vi "Defect Buddy 2014-11-16.vi"() -> ()   [LabVIEW 2010]
uses:
  <vilib>/addons/database/_DB Variant To Data/Database Variant To Data.xnode
  <vilib>/addons/database/NI_Database_API.lvlib
  <vilib>/picture/3D Picture Control/NI_3D Picture Control.lvlib
  <vilib>/Utility/file.llb/Write To Spreadsheet File (string).vi
  <vilib>/addons/database/Connection.llb/Conn Execute.vi
  <vilib>/addons/database/Recordset.llb/Rec Destroy - Connection.vi
  <vilib>/addons/database/Recordset.llb/Rec Fetch Recordset Data (R).vi
  <vilib>/addons/database/Connection.llb/DB Tools Open Connec (Path).vi
  <vilib>/addons/database/Connection.llb/Conn ObjectReference.ctl
panel:
  out "Separate Defects":cluster{i32, i32}[](array[cluster])
  in  "Bound Pairs":T1(array[cluster])
  out "element 2":cluster{i32, i32}
  out "element":cluster{i32, i32}
  out "Array 2":T2(array[cluster])
  out "Array":string[][](array[string])
  out "spreadsheet string":string
  in  "Volumes":dbl[](array[numeric])=[5230.5515143, 4360.60278, 2309.371815, 7792.576126]
  in  "Markov-Payne Correction":bool
  out "Loaded Structure":T3={"Structure Name"="Batch6_3+111 Quasi-Bulk", "Lattice vector a"=[9.1641, 0.0, 0.0], "Lattice vector b"=[0.0, 7.93635, 0.0], "Lattice vector c"=[0.0, 0.0, 53.7091], "Atoms Array"=[{"Atom Name"="", "Positions (Direct)"=[[0.036896, 0.129554, 0.035254], [0.536896, 0.129554, 0.035254], [0.286896, 0.629554, 0.035254], [0.786896, 0.629554, 0.035254], [0.285415, 0.295133, 0.107673], [0.785415, 0.295133, 0.107673], [0.035415, 0.795133, 0.107673], [0.535415, 0.795133, 0.107673], [0.033615, 0.463308, 0.180101], [0.533615, 0.463308, 0.180101], [0.283615, 0.963308, 0.180101], [0.783615, 0.963308, 0.180101], [0.030844, 0.131453, 0.252535], [0.530844, 0.131453, 0.252535], [0.280844, 0.631453, 0.252535], [0.780844, 0.631453, 0.252535], [0.278379, 0.302058, 0.324923], [0.778379, 0.302058, 0.324923], [0.028379, 0.802058, 0.324923], [0.528379, 0.802058, 0.324923], [0.031198, 0.471844, 0.397363], [0.531198, 0.471844, 0.397363], [0.281198, 0.971844, 0.397363], [0.781198, 0.971844, 0.397363], [0.03247, 0.140643, 0.469814], [0.53247, 0.140643, 0.469814], [0.28247, 0.640643, 0.469814], [0.78247, 0.640643, 0.469814], [0.284308, 0.303948, 0.542263], [0.784308, 0.303948, 0.542263], [0.034308, 0.803948, 0.542263], [0.534308, 0.803948, 0.542263], [0.035944, 0.468219, 0.614701], [0.535944, 0.468219, 0.614701], [0.285944, 0.968219, 0.614701], [0.785944, 0.968219, 0.614701], [0.037813, 0.131858, 0.687216], [0.537813, 0.131858, 0.687216], [0.787813, 0.631858, 0.687216], [0.287813, 0.631858, 0.687216], [0.038238, 0.463759, 0.759817], [0.538238, 0.463759, 0.759817], [0.288238, 0.963758, 0.759817], [0.788238, 0.963758, 0.759817], [0.038639, 0.130134, 0.831025], [0.538639, 0.130134, 0.831025], [0.288639, 0.630134, 0.831025], [0.788639, 0.630134, 0.831025], [0.285712, 0.295024, 0.89873], [0.785712, 0.295024, 0.89873], [0.035712, 0.795024, 0.89873], [0.535712, 0.795024, 0.89873], [0.032596, 0.464879, 0.966384], [0.532596, 0.464879, 0.966384], [0.282596, 0.964879, 0.966384], [0.782596, 0.964879, 0.966384]], "Positions (Cartesian)"=[[0.33811863359999994, 1.0281858879, 1.8934606114], [4.9201686336, 1.0281858879, 1.8934606114], [2.6291436335999996, 4.9963608879, 1.8934606114], [7.2111936336, 4.9963608879, 1.8934606114], [2.6155716014999997, 2.34227878455, 5.7830199243000004], [7.197621601499999, 2.34227878455, 5.7830199243000004], [0.3245466015, 6.31045378455, 5.7830199243000004], [4.9065966014999995, 6.31045378455, 5.7830199243000004], [0.30805122149999997, 3.6769744458, 9.673062619100001], [4.890101221499999, 3.6769744458, 9.673062619100001], [2.5990762215, 7.6451494458, 9.673062619100001], [7.1811262215, 7.6451494458, 9.673062619100001], [0.2826575004, 1.04325701655, 13.5634275685], [4.8647075004, 1.04325701655, 13.5634275685], [2.5736825004, 5.011432016550001, 13.5634275685], [7.155732500399999, 5.011432016550001, 13.5634275685], [2.5510929938999998, 2.3972380083, 17.4513218993], [7.1331429939, 2.3972380083, 17.4513218993], [0.2600679939, 6.3654130083, 17.4513218993], [4.8421179939000005, 6.3654130083, 17.4513218993], [0.28590159179999997, 3.7447191294, 21.3420091033], [4.867951591799999, 3.7447191294, 21.3420091033], [2.5769265918, 7.7128941294, 21.3420091033], [7.158976591799999, 7.7128941294, 21.3420091033], [0.29755832699999996, 1.11619207305, 25.2332871074], [4.879608327, 1.11619207305, 25.2332871074], [2.588583327, 5.08436707305, 25.2332871074], [7.170633327, 5.08436707305, 25.2332871074], [2.6054269428, 2.4122377098, 29.124457693300002], [7.1874769428, 2.4122377098, 29.124457693300002], [0.31440194279999994, 6.3804127098, 29.124457693300002], [4.8964519428, 6.3804127098, 29.124457693300002], [0.32939441039999995, 3.71594986065, 33.0150374791], [4.9114444104, 3.71594986065, 33.0150374791], [2.6204194104, 7.684124860650001, 33.0150374791], [7.202469410399999, 7.684124860650001, 33.0150374791], [0.3465221133, 1.0464712383, 36.909752865600005], [4.9285721133, 1.0464712383, 36.909752865600005], [7.2195971133, 5.0146462383, 36.909752865600005], [2.6375471132999997, 5.0146462383, 36.909752865600005], [0.3504168558, 3.6805537396499997, 40.809087234699994], [4.9324668557999995, 3.6805537396499997, 40.809087234699994], [2.6414418557999997, 7.6487208033, 40.809087234699994], [7.2234918558, 7.6487208033, 40.809087234699994], [0.35409165989999997, 1.0327889709, 44.6336048275], [4.9361416599, 1.0327889709, 44.6336048275], [2.6451166599, 5.0009639709, 44.6336048275], [7.227166659899999, 5.0009639709, 44.6336048275], [2.6182933392, 2.3414137224, 48.269979443000004], [7.200343339199999, 2.3414137224, 48.269979443000004], [0.3272683392, 6.3095887224, 48.269979443000004], [4.9093183391999995, 6.3095887224, 48.269979443000004], [0.29871300359999997, 3.6894424516499997, 51.9036148944], [4.880763003599999, 3.6894424516499997, 51.9036148944], [2.5897380036, 7.65761745165, 51.9036148944], [7.171788003599999, 7.65761745165, 51.9036148944]]}, {"Atom Name"="", "Positions (Direct)"=[[0.286795, 0.296109, 0.054458], [0.786795, 0.296109, 0.054458], [0.036795, 0.796109, 0.054458], [0.536795, 0.796109, 0.054458], [0.035258, 0.462031, 0.126878], [0.535258, 0.462031, 0.126878], [0.285258, 0.962031, 0.126878], [0.785258, 0.962031, 0.126878], [0.033445, 0.130094, 0.199309], [0.533445, 0.130094, 0.199309], [0.283445, 0.630094, 0.199309], [0.783445, 0.630094, 0.199309], [0.280766, 0.298203, 0.27171], [0.780766, 0.298203, 0.27171], [0.030766, 0.798203, 0.27171], [0.530766, 0.798203, 0.27171], [0.028505, 0.468822, 0.344121], [0.528505, 0.468822, 0.344121], [0.278505, 0.968822, 0.344121], [0.778505, 0.968822, 0.344121], [0.03126, 0.138635, 0.416572], [0.53126, 0.138635, 0.416572], [0.28126, 0.638635, 0.416572], [0.78126, 0.638635, 0.416572], [0.282556, 0.307128, 0.489026], [0.782556, 0.307128, 0.489026], [0.032556, 0.807128, 0.489026], [0.532556, 0.807128, 0.489026], [0.034374, 0.470438, 0.56147], [0.534374, 0.470438, 0.56147], [0.284374, 0.970438, 0.56147], [0.784374, 0.970438, 0.56147], [0.035964, 0.134698, 0.633895], [0.535964, 0.134698, 0.633895], [0.285964, 0.634698, 0.633895], [0.785964, 0.634698, 0.633895], [0.037794, 0.465111, 0.706493], [0.537794, 0.465111, 0.706493], [0.787794, 0.965111, 0.706493], [0.287794, 0.965111, 0.706493], [0.038181, 0.130274, 0.779081], [0.538181, 0.130274, 0.779081], [0.288181, 0.630273, 0.779081], [0.788181, 0.630273, 0.779081], [0.288548, 0.296604, 0.847022], [0.788548, 0.296604, 0.847022], [0.038548, 0.796604, 0.847022], [0.538548, 0.796604, 0.847022], [0.035661, 0.461866, 0.914714], [0.535661, 0.461866, 0.914714], [0.285661, 0.961866, 0.914714], [0.785661, 0.961866, 0.914714], [0.032517, 0.131341, 0.982331], [0.532517, 0.131341, 0.982331], [0.282517, 0.631341, 0.982331], [0.782517, 0.631341, 0.982331]], "Positions (Cartesian)"=[[2.6282180595, 2.35002466215, 2.9248901678], [7.2102680595, 2.35002466215, 2.9248901678], [0.3371930595, 6.31819966215, 2.9248901678], [4.9192430595, 6.31819966215, 2.9248901678], [0.32310783779999996, 3.66683972685, 6.814503189799999], [4.9051578378, 3.66683972685, 6.814503189799999], [2.6141328378, 7.63501472685, 6.814503189799999], [7.1961828377999995, 7.63501472685, 6.814503189799999], [0.3064933245, 1.0324715168999998, 10.704707011899998], [4.8885433245, 1.0324715168999998, 10.704707011899998], [2.5975183244999998, 5.000646516900001, 10.704707011899998], [7.179568324499999, 5.000646516900001, 10.704707011899998], [2.5729677006, 2.36664337905, 14.593299561], [7.155017700599999, 2.36664337905, 14.593299561], [0.2819427006, 6.33481837905, 14.593299561], [4.863992700599999, 6.33481837905, 14.593299561], [0.2612226705, 3.7207354797, 18.4824292011], [4.843272670499999, 3.7207354797, 18.4824292011], [2.5522476705, 7.6889104797, 18.4824292011], [7.1342976705, 7.6889104797, 18.4824292011], [0.286469766, 1.1002558822500002, 22.3737072052], [4.8685197659999995, 1.1002558822500002, 22.3737072052], [2.577494766, 5.0684308822499995, 22.3737072052], [7.159544765999999, 5.0684308822499995, 22.3737072052], [2.5893714396, 2.4374753028000002, 26.2651463366], [7.1714214396, 2.4374753028000002, 26.2651463366], [0.2983464396, 6.4056503028, 26.2651463366], [4.8803964396, 6.4056503028, 26.2651463366], [0.3150067734, 3.7335606213, 30.156048377], [4.8970567734, 3.7335606213, 30.156048377], [2.6060317734, 7.7017356213, 30.156048377], [7.1880817733999995, 7.7017356213, 30.156048377], [0.3295776924, 1.0690104723, 34.045929944499996], [4.9116276924, 1.0690104723, 34.045929944499996], [2.6206026924, 5.0371854723, 34.045929944499996], [7.202652692399999, 5.0371854723, 34.045929944499996], [0.3463479954, 3.69128368485, 37.9451031863], [4.928397995399999, 3.69128368485, 37.9451031863], [7.2194229953999995, 7.659458684850001, 37.9451031863], [2.6373729954, 7.659458684850001, 37.9451031863], [0.34989450209999995, 1.0339000599000001, 41.843739337100004], [4.9319445020999995, 1.0339000599000001, 41.843739337100004], [2.6409195021, 5.00206712355, 41.843739337100004], [7.2229695021, 5.00206712355, 41.843739337100004], [2.6442827268, 2.3539531553999997, 45.4927893002], [7.2263327268, 2.3539531553999997, 45.4927893002], [0.35325772679999995, 6.3221281554, 45.4927893002], [4.9353077268, 6.3221281554, 45.4927893002], [0.3268009701, 3.6655302291, 49.1284656974], [4.9088509701000005, 3.6655302291, 49.1284656974], [2.6178259700999997, 7.6337052291, 49.1284656974], [7.1998759701, 7.6337052291, 49.1284656974], [0.29798903969999996, 1.04236814535, 52.760113912099996], [4.8800390397, 1.04236814535, 52.760113912099996], [2.5890140397, 5.010543145350001, 52.760113912099996], [7.1710640397, 5.010543145350001, 52.760113912099996]]}], "# of atoms"=112}
  out "Indicies":cluster{i32, i32}[](array[cluster])
  out "All Hosts and Defects":T4(array[cluster])
  out "Thermodynamic Fermi Level (eV)":dbl
  out "Defects to Bind":i32[](array[numeric])
  in  "Plot Binding Energy":bool
  in  "Calc Thermodynamic Fermi Level":bool
  in  "Thermodynamic Fermi Level":i32
  in  "Color Array Type":T5(ring)=enum."Contrasting Colors"
  in  "Show Charge Transitions":bool=TRUE
  out "connection reference":T6
  in  "Plots Tab":T7(tab)
  in  "Make Awesome Looking":bool
  out "Te Rich Limit":cluster{dbl[], dbl[]}[](graph)
  out "Cd Rich Limit":cluster{"appended array":dbl[], dbl[]}[](graph)
  in  "Chemical Potential":dbl(slide) scale=0.0..1.0
  in  "Chemical Potential 2":dbl(slide)=1.0 scale=0.0..1.0
  in  "Save as a table":bool
  out "Te Rich Limit 2":cluster{dbl[], dbl[]}[](graph)
  out "Cd Rich Limit 2":cluster{"appended array":dbl[], dbl[]}[](graph)
  in  "Chemical Potential 5":dbl(slide) scale=0.0..1.0
  in  "Chemical Potential 3":dbl(slide)=1.0 scale=0.0..1.0
  in  "Save as a table 2":bool
  in  "Bound Pairs List":i32[](listbox)
  in  "Assign Bound Calculation":bool
  in  "Seperate Defects":i32(listbox)
  in  "Set as seperate defects":bool
  out "Binding Energy":cluster{"Array":dbl[], dbl[]}[](graph)
  in  "Binding Energy Chem Pot":dbl(slide) scale=0.0..1.0
  out "Defect Energy Levels":cluster{dbl[], dbl[]}[](graph)
  in  "Buckets":string[][](array[combo])
  out "Atomic Structure":refnum<vi>(3d-picture)
  in  "Load in VESTA":bool
  in  "Atomic Structures":i32(listbox)
  in  "Options":cluster{"Border?":bool, "Bonds?":bool}
  in  "Atom Size":dbl=0.75
  in  "Plot Atomic Structure":bool
  in  "Scale":dbl(slide)=0.07482993197278912 scale=0.0..0.5
  in  "Setup Camera":bool
  in  "Ignore Location":bool
  in  "Potential Re-alignment":bool
  out "Defects":T8(array[cluster])
  out "Base Object":refnum<vi>
  in  "VBM":dbl=1.79581
  in  "Pure Structures with defects":i32[](listbox)
  in  "Related Defects":i32[](listbox)
  in  "UDL":path=path "D:/Ab-initio/VASP Calcs/VASP DB.udl"
  # "Cd Rich"
  # "Te Rich"
  # "Cd Rich"
  # "Te Rich"
  # "p-type"
  # "n-type"
  # "p-type"
  # "n-type"
  # "Cd Rich"
  # "Te Rich"
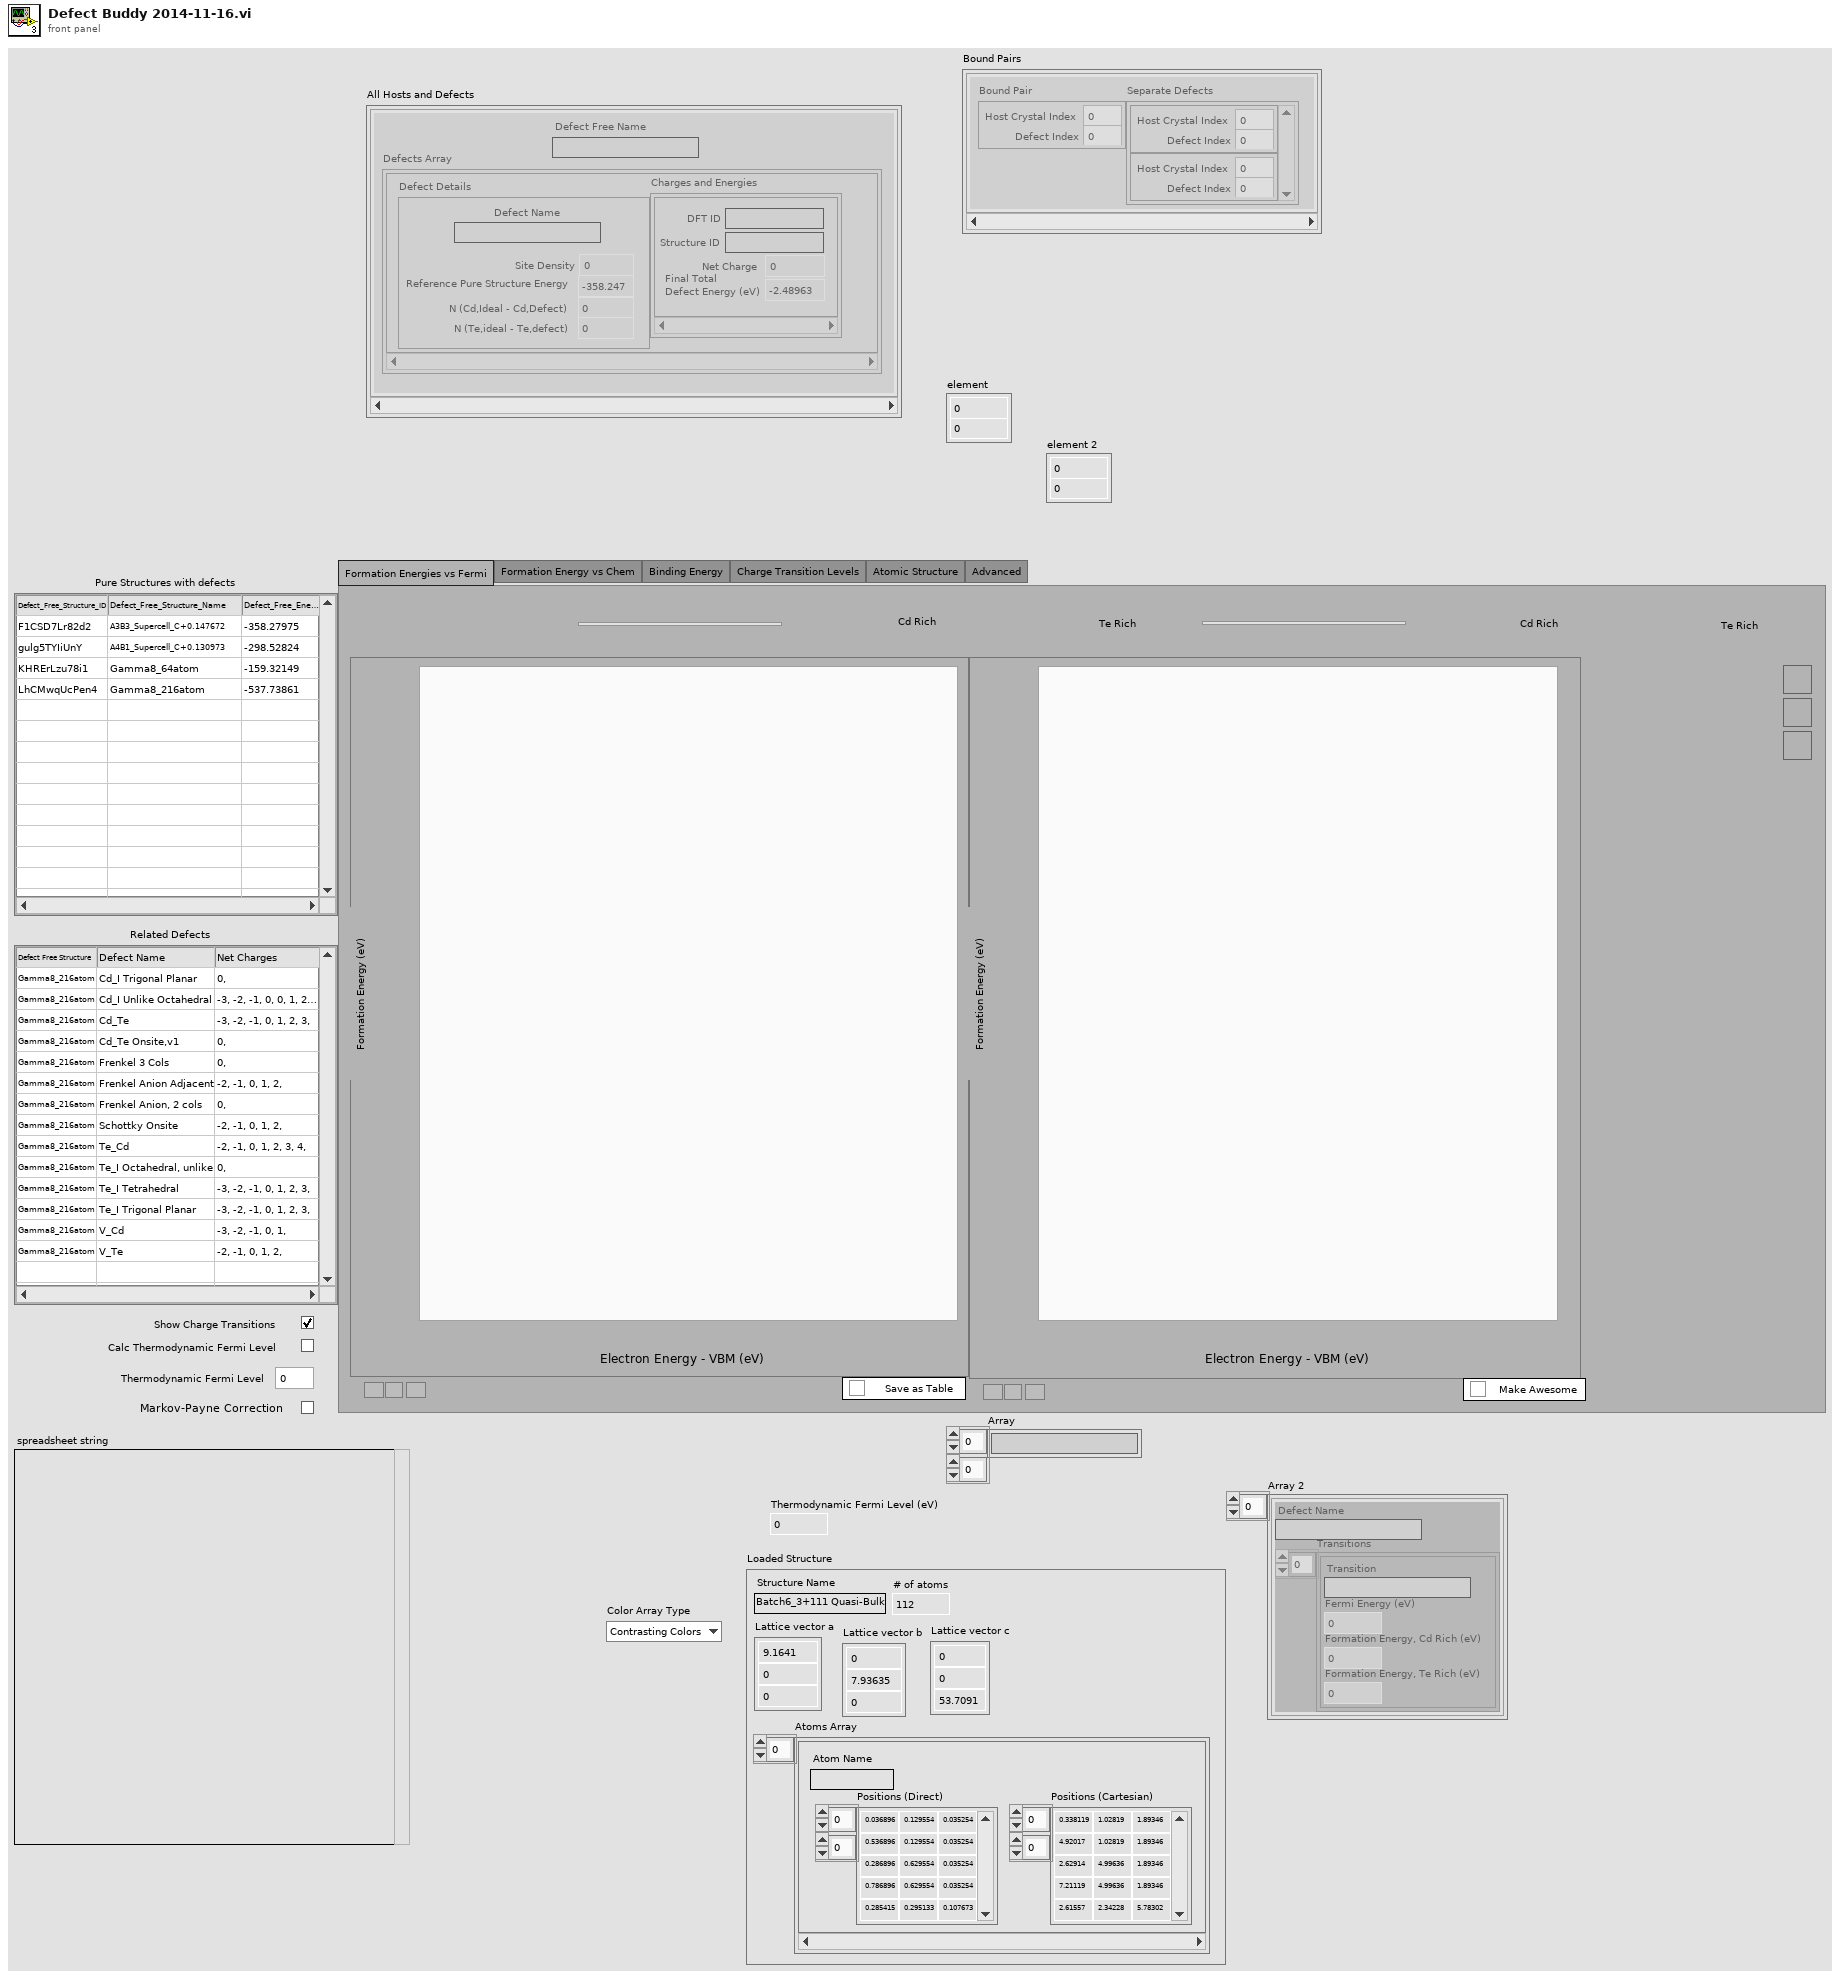
[diagram p1: front panel]
types:
  T1 = cluster{"Bound Pair":cluster{"Host Crystal Index":i32, "Defect Index":i32}, "Separate Defects":cluster{"Host Crystal Index":i32, "Defect Index":i32}[]}[]
  T2 = cluster{"Defect Name":string, "Transitions":cluster{"Transition":string, "Fermi Energy (eV)":dbl, "Formation Energy, Cd Rich (eV)":dbl, "Formation Energy, Te Rich (eV)":dbl}[]}[]
  T3 = cluster{"Structure Name":string, "Lattice vector a":dbl[], "Lattice vector b":dbl[], "Lattice vector c":dbl[], "Atoms Array":cluster{"Atom Name":string, "Positions (Direct)":dbl[][], "Positions (Cartesian)":dbl[][]}[], "# of atoms":i32}
  T4 = cluster{"Defect Free Name":string, "Defects Array":cluster{"Defect Details":cluster{"Defect Name":string, "Site Density":dbl, "Reference Pure Structure Energy":dbl, "N (Cd,Ideal - Cd,Defect)":i32, "N (Te,ideal - Te,defect)":i32}, "Charges and Energies":cluster{"DFT ID":string, "Structure ID":string, "Net Charge":i32, "Final Total \nDefect Energy (eV)":dbl}[]}[]}[]
  T5 = enum16{"Visible Spectrum", "Greyscale", "Contrasting Colors"}
  T6 = typedef "NI_Database_API.lvlib/Conn ObjectReference.ctl" = refnum<k1>
  T7 = enum32{"Formation Energies vs Fermi", "Formation Energy vs Chem", "Binding Energy", "Charge Transition Levels", "Atomic Structure", "Advanced"}
  T8 = cluster{"Defect Details":cluster{"Defect Name":string, "Site Density":dbl, "Reference Pure Structure Energy":dbl, "N (Cd,Ideal - Cd,Defect)":i32, "N (Te,ideal - Te,defect)":i32}, "Charges and Energies":cluster{"Net Charge":i32, "Final Total \nDefect Energy (eV)":dbl}[]}[]
  T9 = typedef "NI_Database_API.lvlib/Rec ObjectReference.ctl" = refnum<k1>
  T10 = cluster{"Name":string, "Color":u32, "Style":u8, "Point Style":u8, "Name Visible":bool, "Allow Drag":bool, "Annotation Mode":u32, "Plot":i32, "Index":i32, "Position":cluster{"X":dbl, "Y":dbl}, "X Scale":u32, "Y Scale":u32, "Show Arrow":bool, "Lock Name":bool, "Plot Area":i32, "Label Offset":cluster{"X":dbl, "Y":dbl}}
  T11 = cluster{"Name":string, "Color":u32, "Style":u8, "Point Style":u8, "Name Visible":bool, "Allow Drag":bool, "Cursor Mode":u32, "Plot":i32, "Index":i32, "Position":cluster{"X":dbl, "Y":dbl}, "X Scale":u32, "Y Scale":u32, "Watch Plots":i32[], "Watch All Plots":bool, "Plot Area":i32, "Label Offset":cluster{"X":dbl, "Y":dbl}}
  T12 = cluster{"Defect Details":cluster{"Defect Name":string, "Site Density":dbl, "Reference Pure Structure Energy":dbl, "N (Cd,Ideal - Cd,Defect)":i32, "N (Te,ideal - Te,defect)":i32}, "Charges and Energies":cluster{"DFT ID":string, "Structure ID":string, "Net Charge":i32, "Final Total \nDefect Energy (eV)":dbl}[]}[]
  T13 = cluster{"Defect Name":string, "Site Density":dbl, "Reference Pure Structure Energy":dbl, "N (Cd,Ideal - Cd,Defect)":i32, "N (Te,ideal - Te,defect)":i32}
  T14 = cluster{"DFT ID":string, "Structure ID":string, "Net Charge":i32, "Final Total \nDefect Energy (eV)":dbl}[]
  T15 = cluster{string, "Defects Array":cluster{"Defect Details":cluster{"Defect Name":string, "Site Density":dbl, "Reference Pure Structure Energy":dbl, "N (Cd,Ideal - Cd,Defect)":i32, "N (Te,ideal - Te,defect)":i32}, "Charges and Energies":cluster{"DFT ID":string, "Structure ID":string, "Net Charge":i32, "Final Total \nDefect Energy (eV)":dbl}[]}[]}
  T16 = cluster{"Name":string, "Color":u32, "Style":u8, "Point Style":u8, "Name Visible":bool, "Allow Drag":bool, "Cursor Mode":u32, "Plot":i32, "Index":i32, "Position":cluster{"X":dbl, "Y":dbl}, "X Scale":u32, "Y Scale":u32, "Watch Plots":i32[], "Watch All Plots":bool, "Plot Area":i32, "Label Offset":cluster{"X":dbl, "Y":dbl}}[]
  T17 = cluster{"Name":string, "Color":u32, "Style":u8, "Point Style":u8, "Name Visible":bool, "Allow Drag":bool, "Annotation Mode":u32, "Plot":i32, "Index":i32, "Position":cluster{"X":dbl, "Y":dbl}, "X Scale":u32, "Y Scale":u32, "Show Arrow":bool, "Lock Name":bool, "Plot Area":i32, "Label Offset":cluster{"X":dbl, "Y":dbl}}[]
  T18 = cluster{"Defect Free Name":string, "Defects Array":cluster{"Defect Details":cluster{"Defect Name":string, "Site Density":dbl, "Reference Pure Structure Energy":dbl, "N (Cd,Ideal - Cd,Defect)":i32, "N (Te,ideal - Te,defect)":i32}, "Charges and Energies":cluster{"DFT ID":string, "Structure ID":string, "Net Charge":i32, "Final Total \nDefect Energy (eV)":dbl}[]}[]}
  T19 = cluster{"Defect Details":cluster{"Defect Name":string, "Site Density":dbl, "Reference Pure Structure Energy":dbl, "N (Cd,Ideal - Cd,Defect)":i32, "N (Te,ideal - Te,defect)":i32}, "Charges and Energies":cluster{"DFT ID":string, "Structure ID":string, "Net Charge":i32, "Final Total \nDefect Energy (eV)":dbl}[]}
  T20 = cluster{"Transition":string, "Fermi Energy (eV)":dbl, "Formation Energy, Cd Rich (eV)":dbl, "Formation Energy, Te Rich (eV)":dbl}[]
  T21 = cluster{"Defect Name":string, "Transitions":cluster{"Transition":string, "Fermi Energy (eV)":dbl, "Formation Energy, Cd Rich (eV)":dbl, "Formation Energy, Te Rich (eV)":dbl}[]}
  T22 = cluster{cluster{i32, i32}, "Separate Defects":cluster{i32, i32}[]}
  T23 = cluster{"Bound Pair":cluster{"Host Crystal Index":i32, "Defect Index":i32}, "Separate Defects":cluster{"Host Crystal Index":i32, "Defect Index":i32}[]}
  T24 = cluster{"Host Crystal Index":i32, "Defect Index":i32}[]
  T25 = cluster{"Lattice vector b[0]":dbl, "Lattice vector b[1]":dbl, "Lattice vector b[2]":dbl}
  T26 = typedef "LVAnnotationListTypeDef.ctl" = cluster{"Name":string, "Color":u32, "Style":u8, "Point Style":u8, "Name Visible":bool, "Allow Drag":bool, "Annotation Mode":u32, "Plot":i32, "Index":i32, "Position":cluster{"X":dbl, "Y":dbl}, "X Scale":u32, "Y Scale":u32, "Show Arrow":bool, "Lock Name":bool, "Plot Area":i32, "Label Offset":cluster{"X":dbl, "Y":dbl}}[]
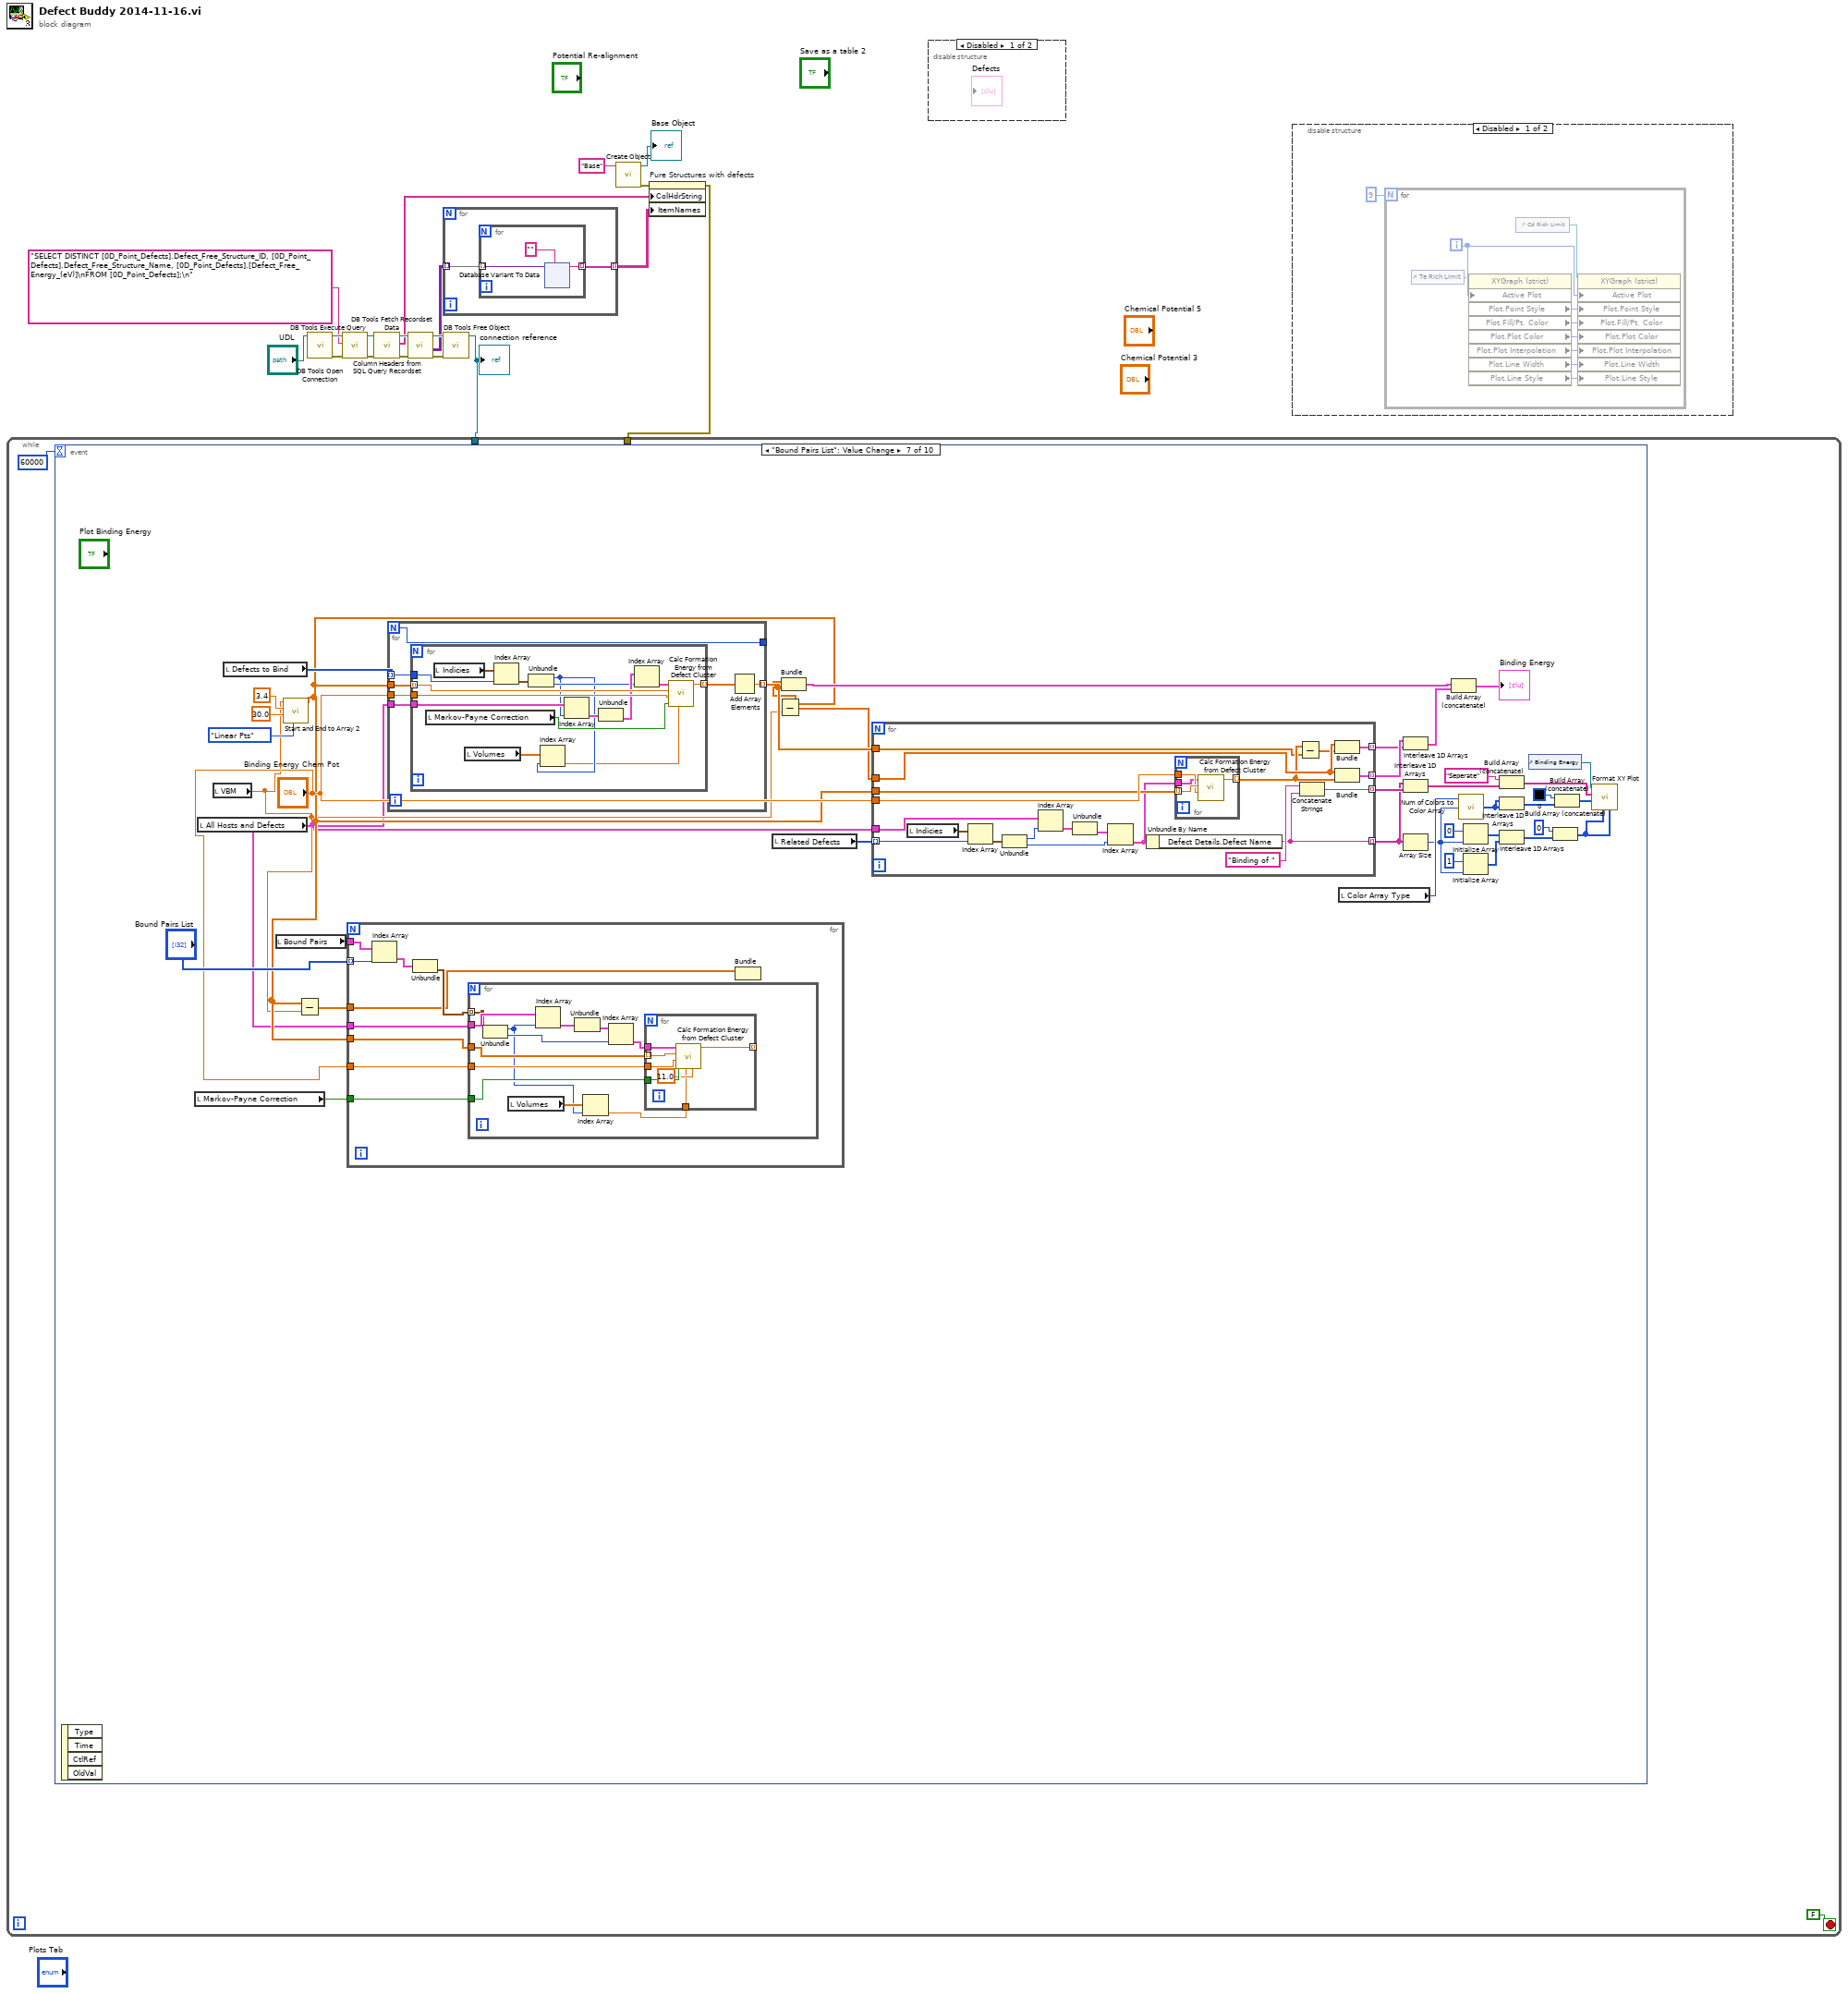
[diagram p0: block diagram]
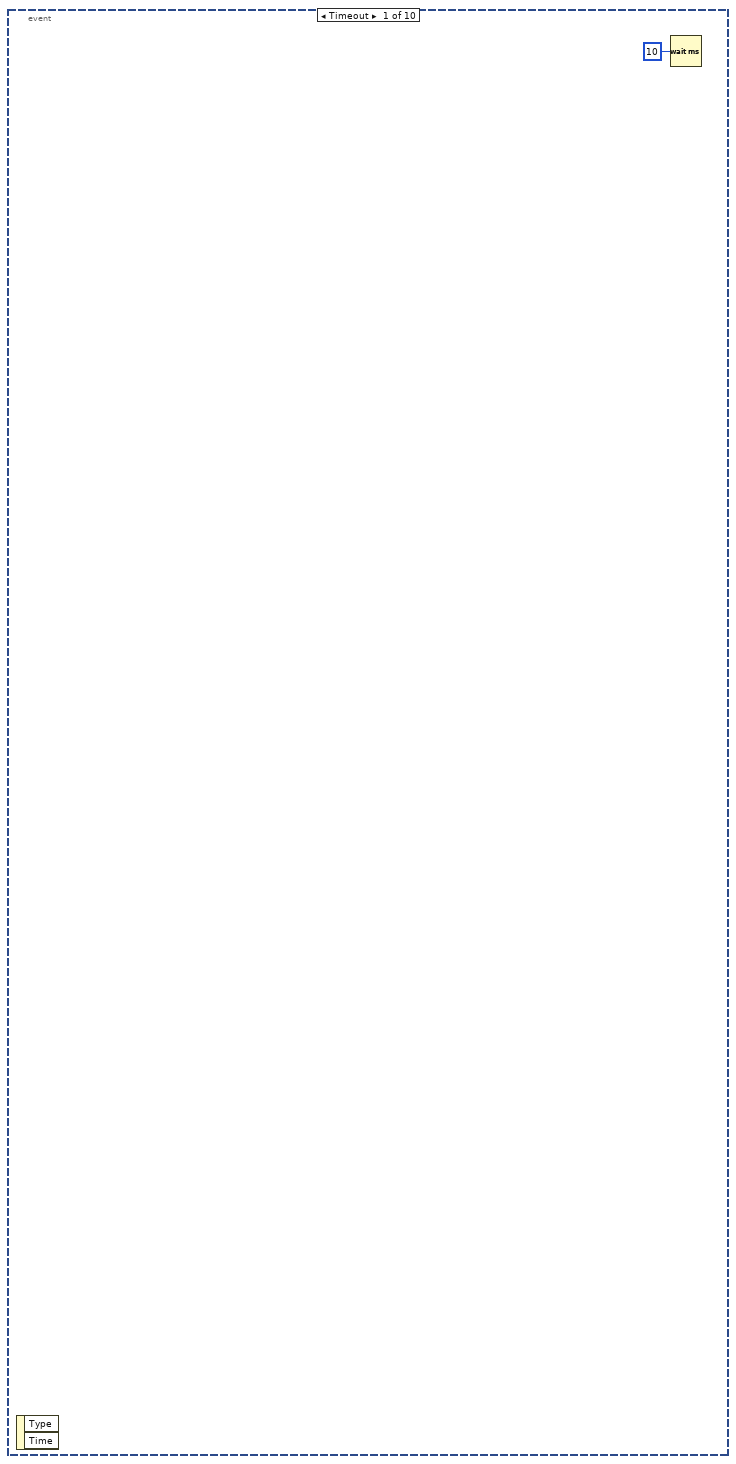
[diagram p4: hidden frame]
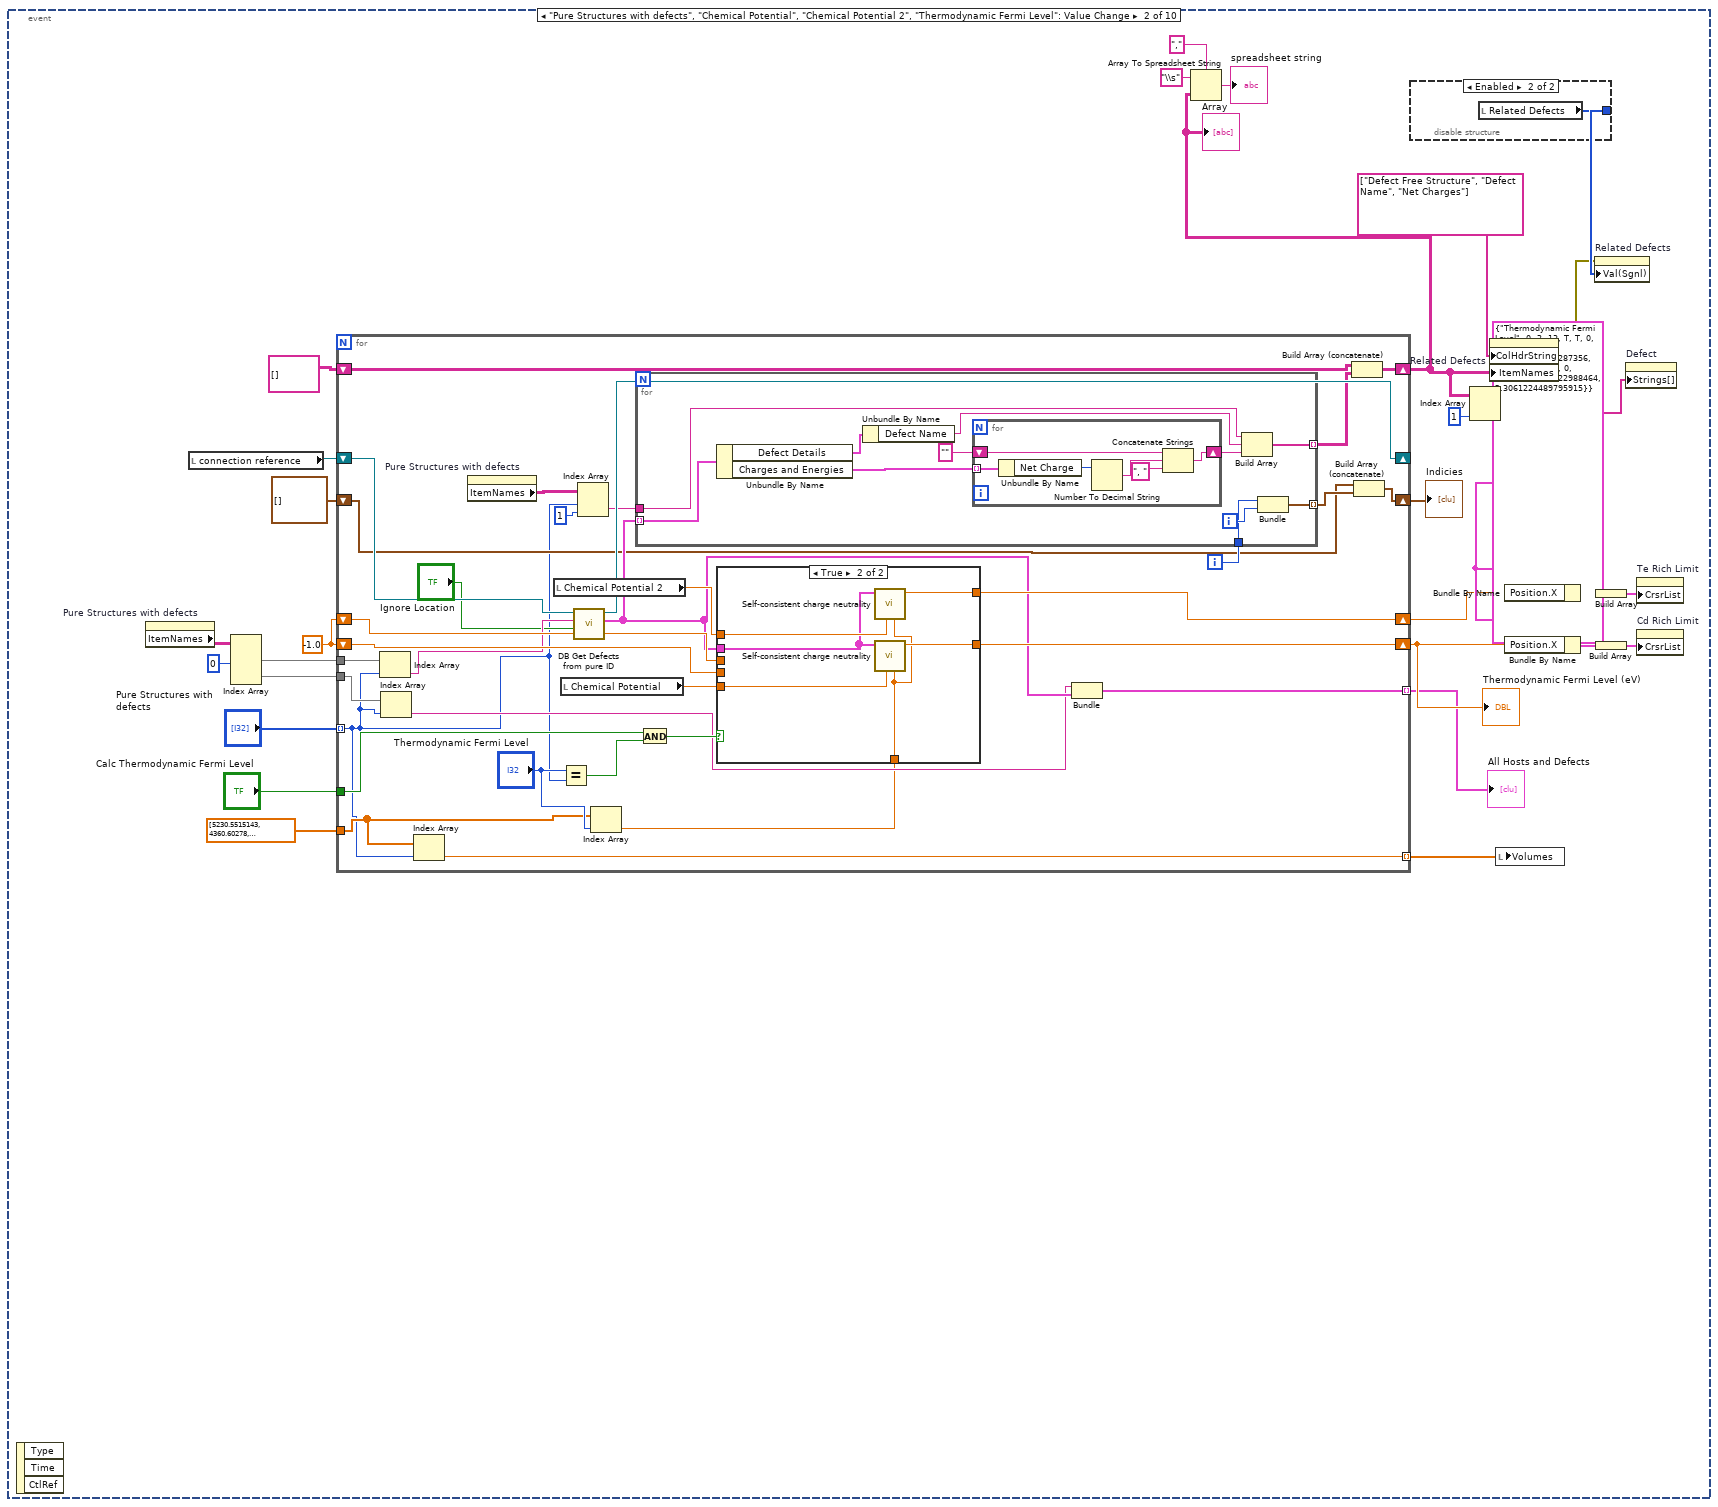
[diagram p5: hidden frame]
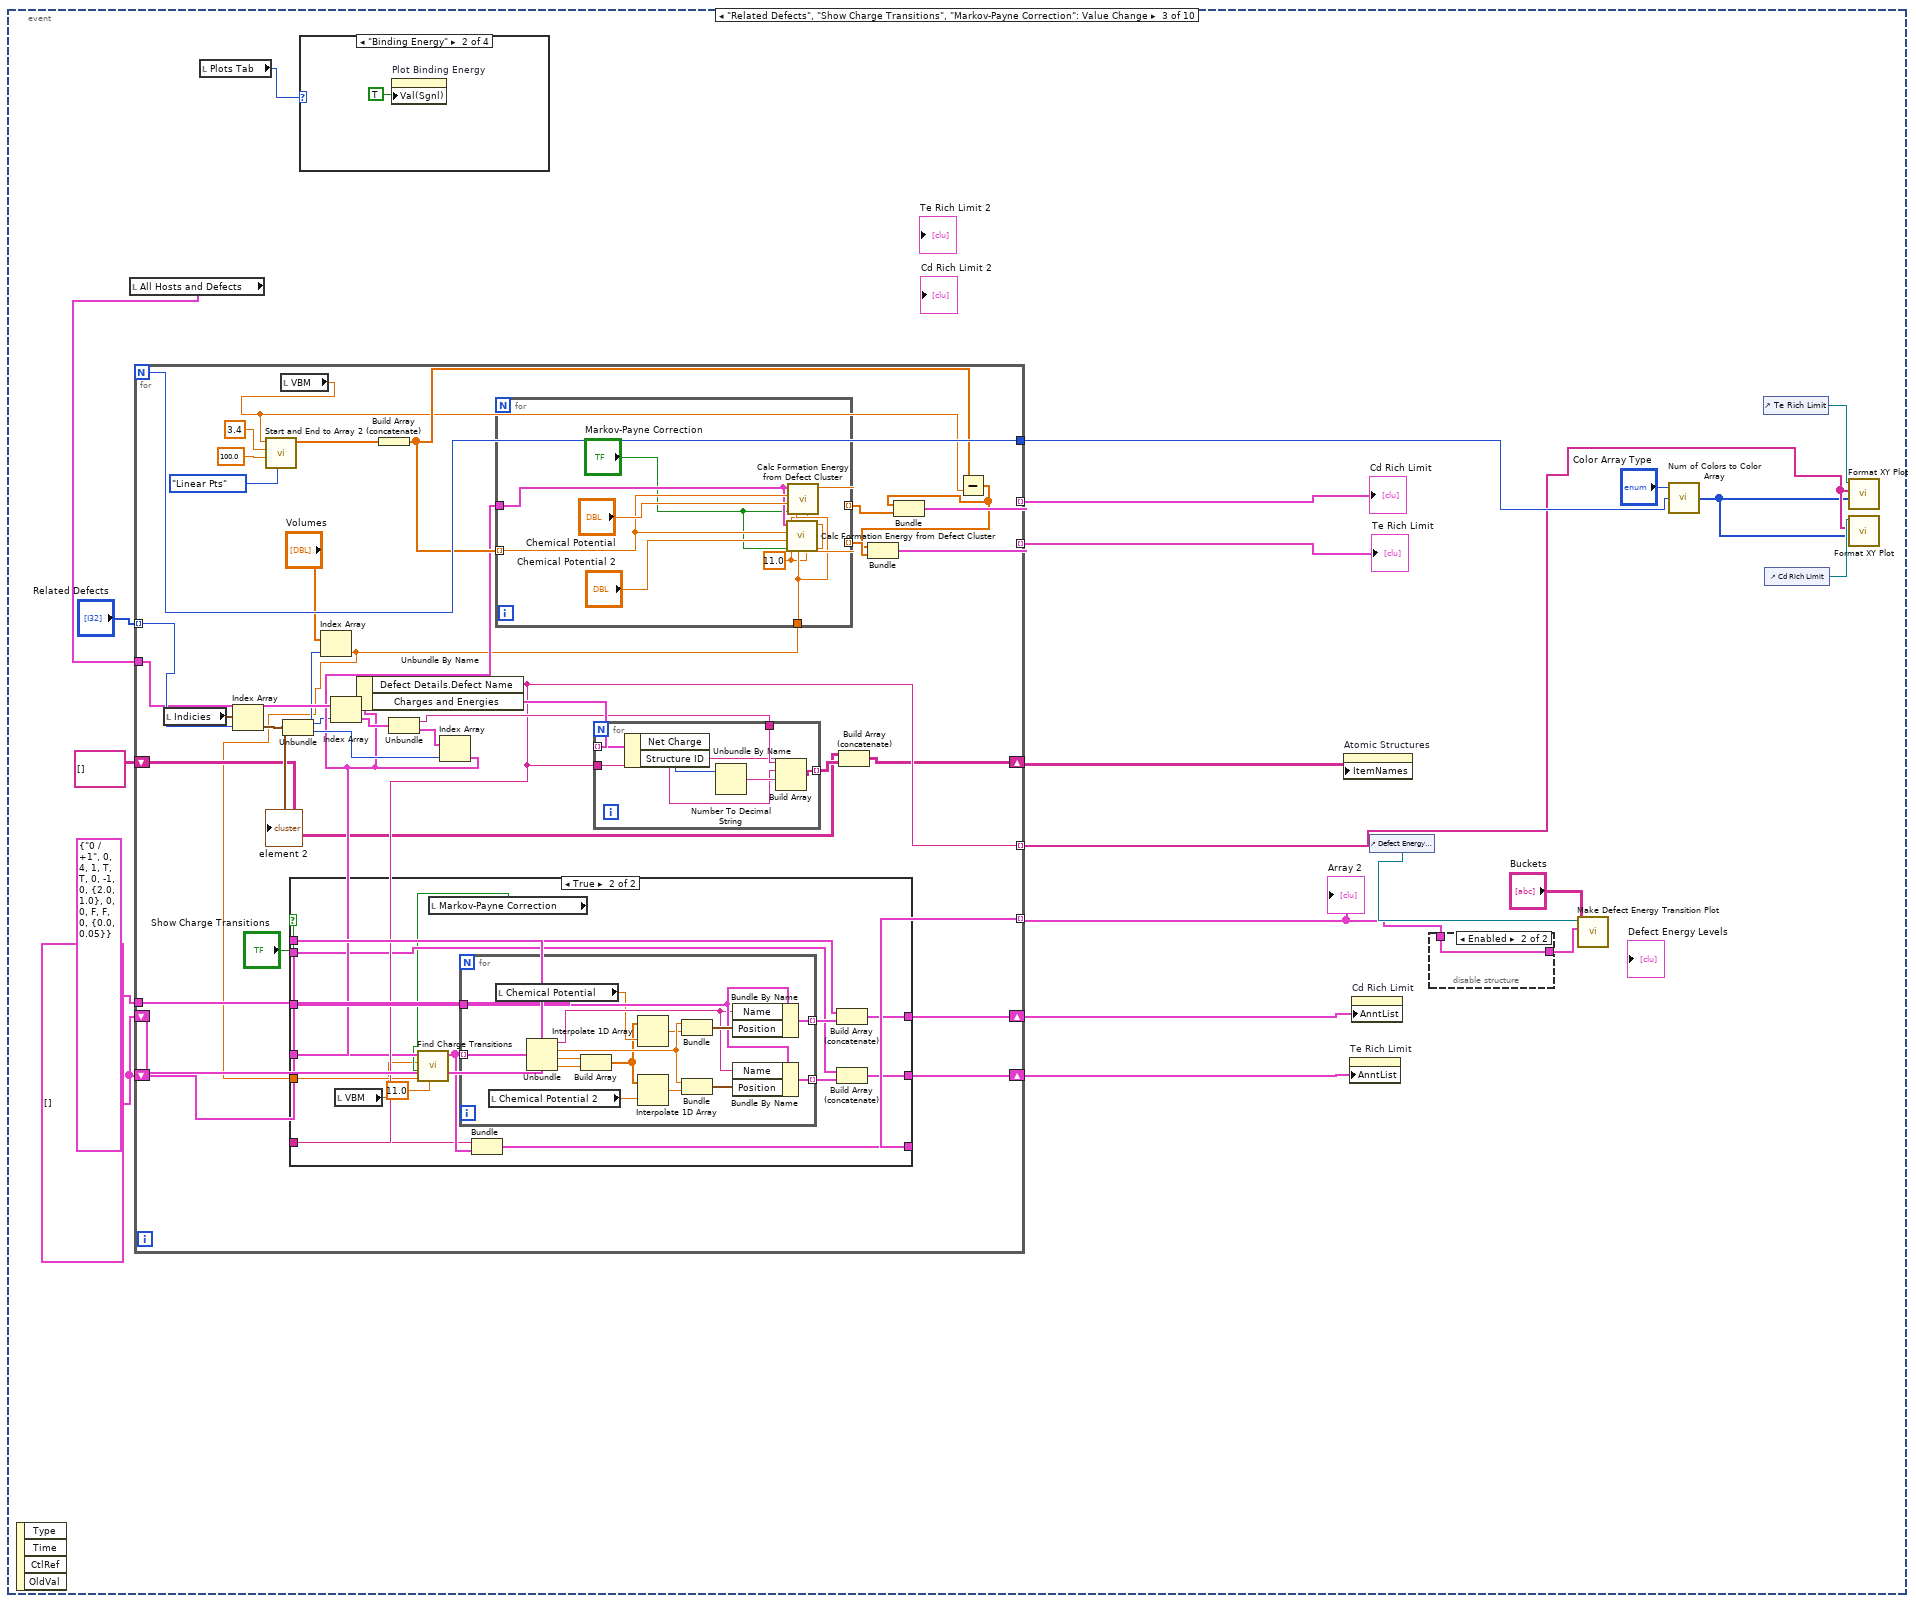
[diagram p8: hidden frame]
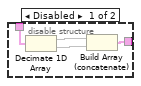
[diagram p9: hidden frame]
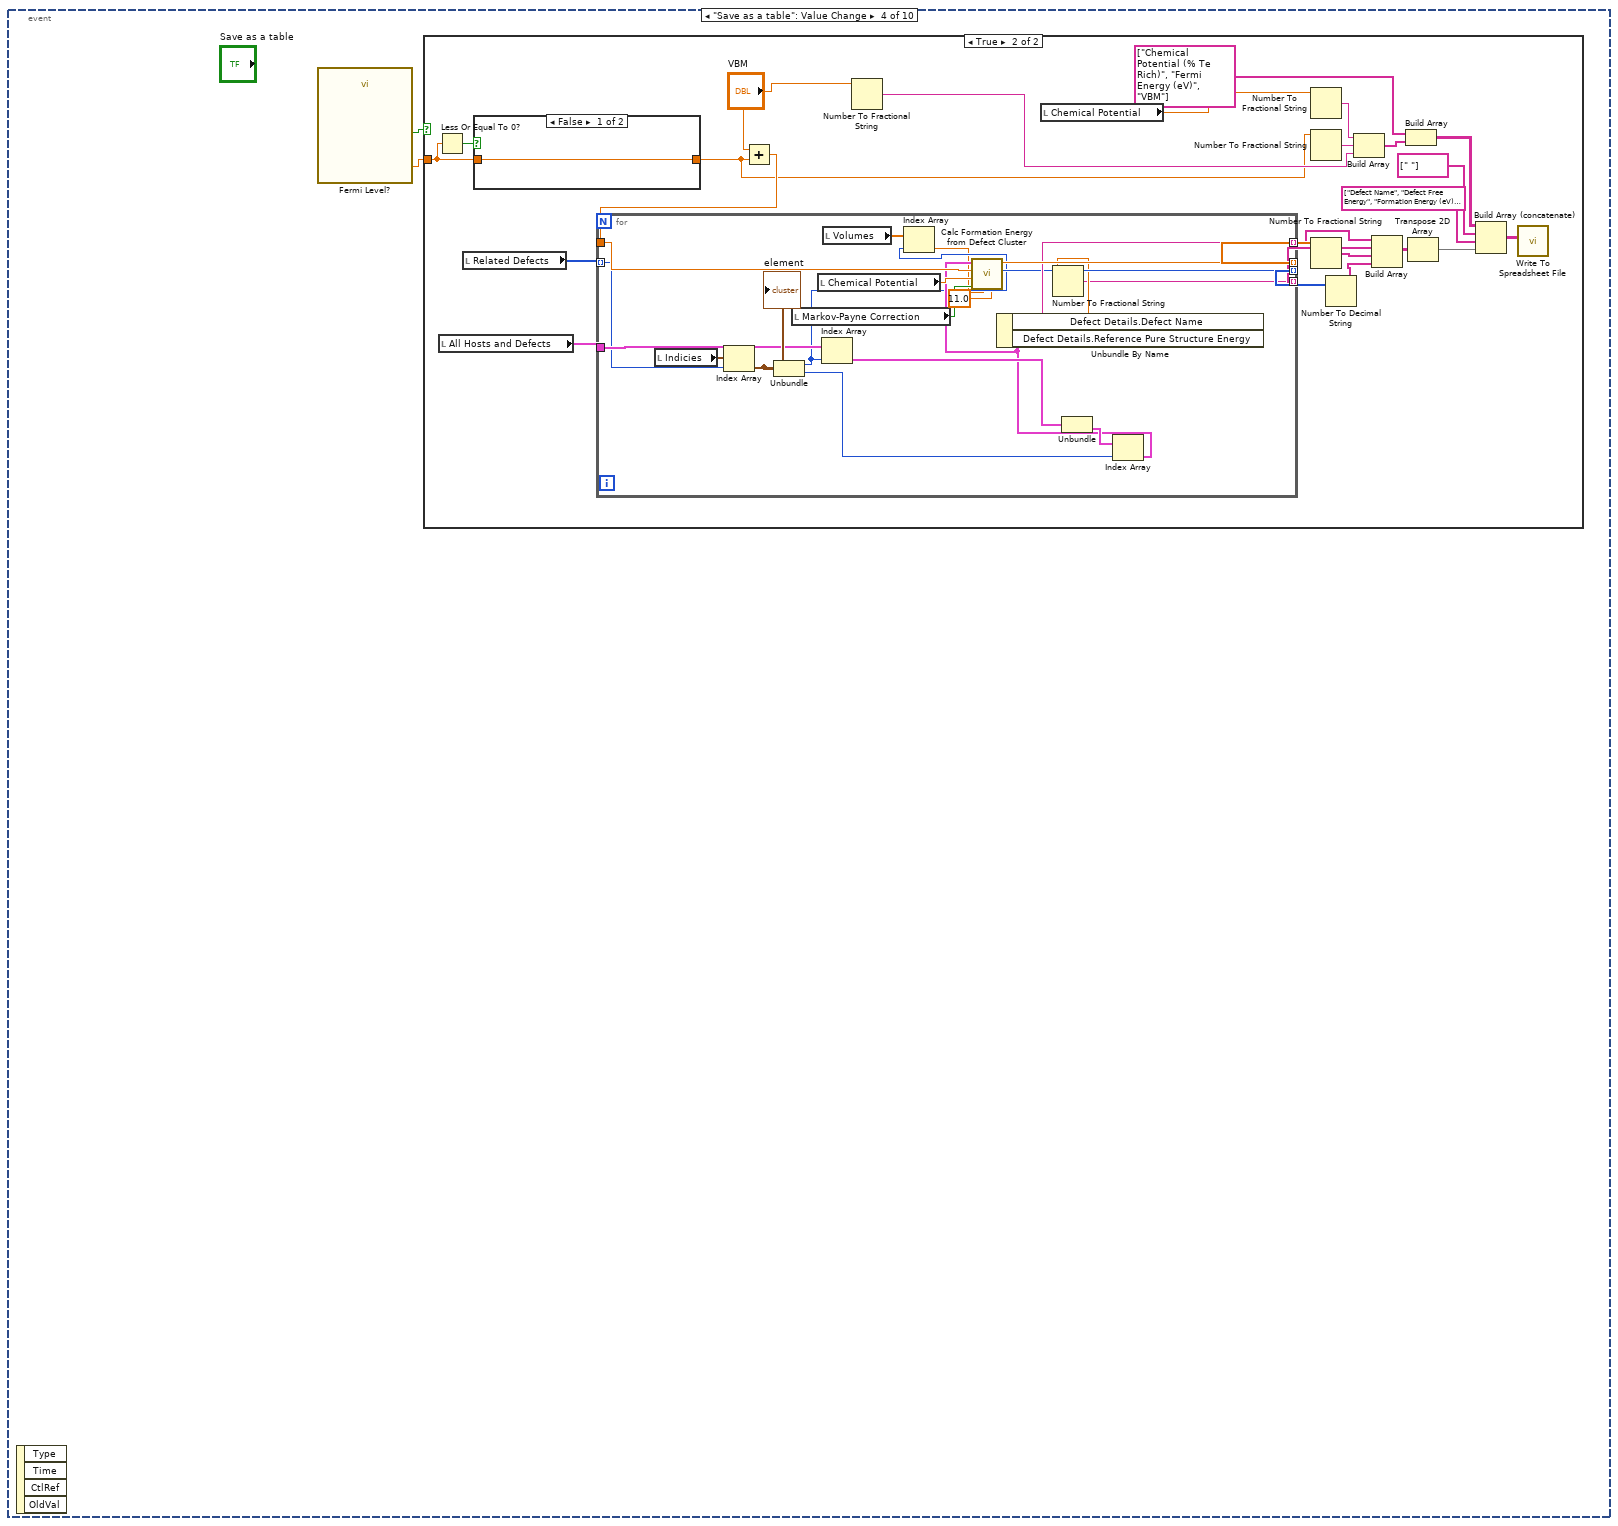
[diagram p14: hidden frame]
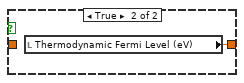
[diagram p16: hidden frame]
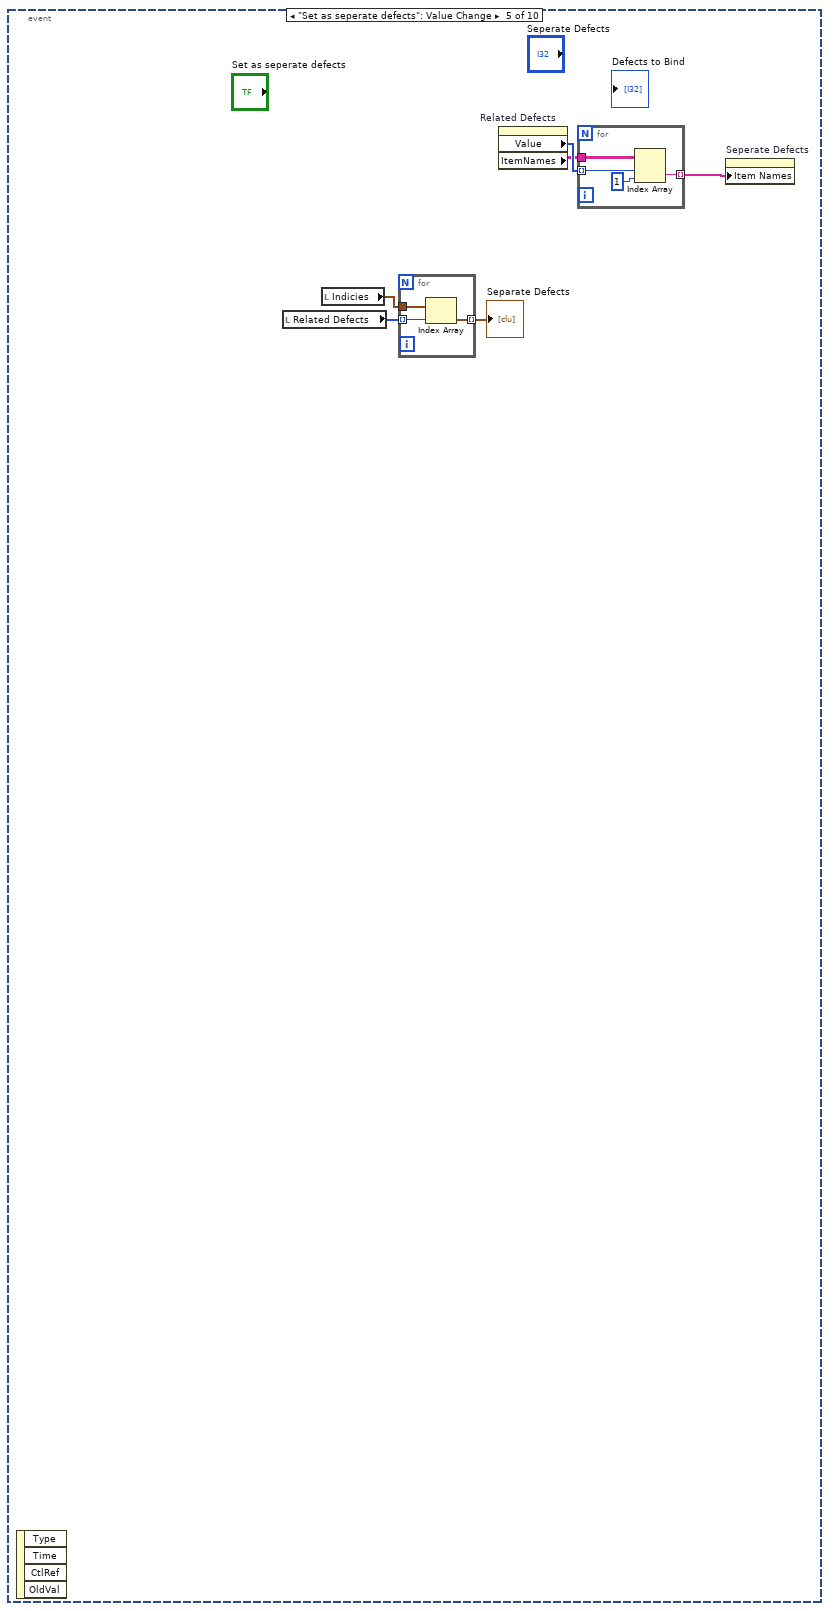
[diagram p17: hidden frame]
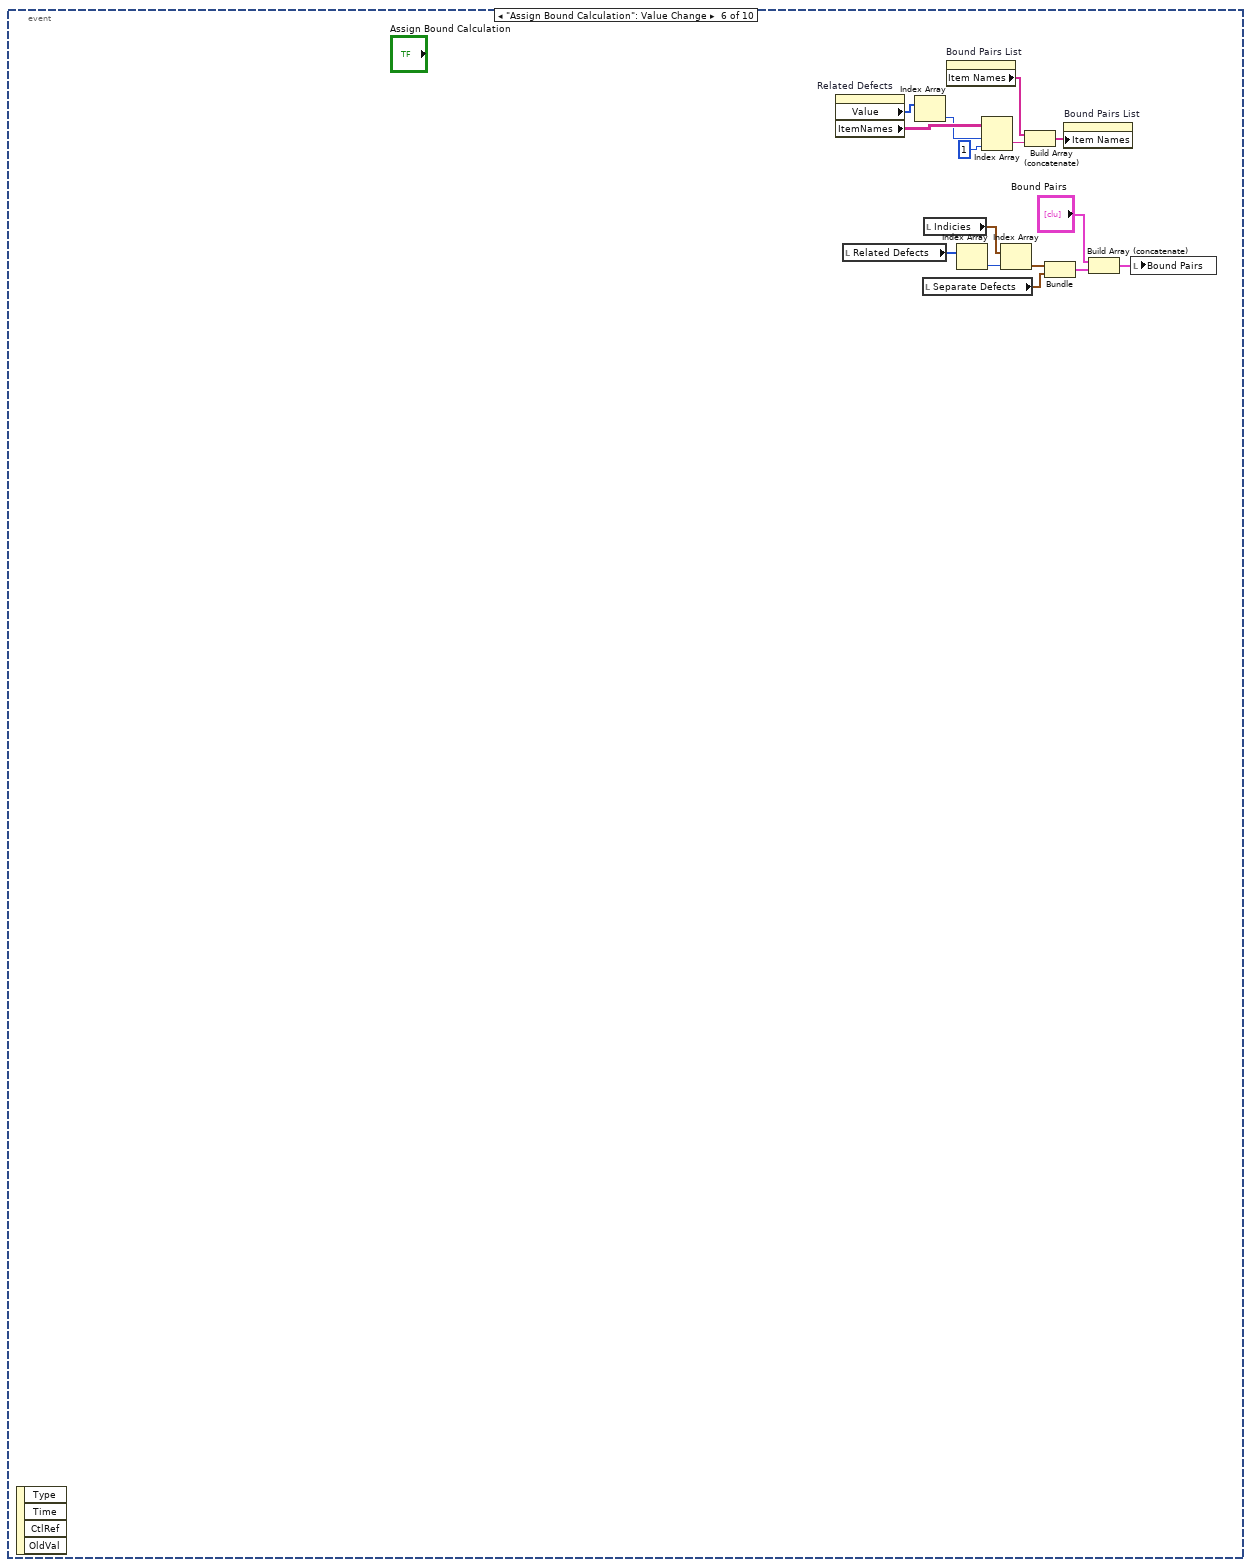
[diagram p18: hidden frame]
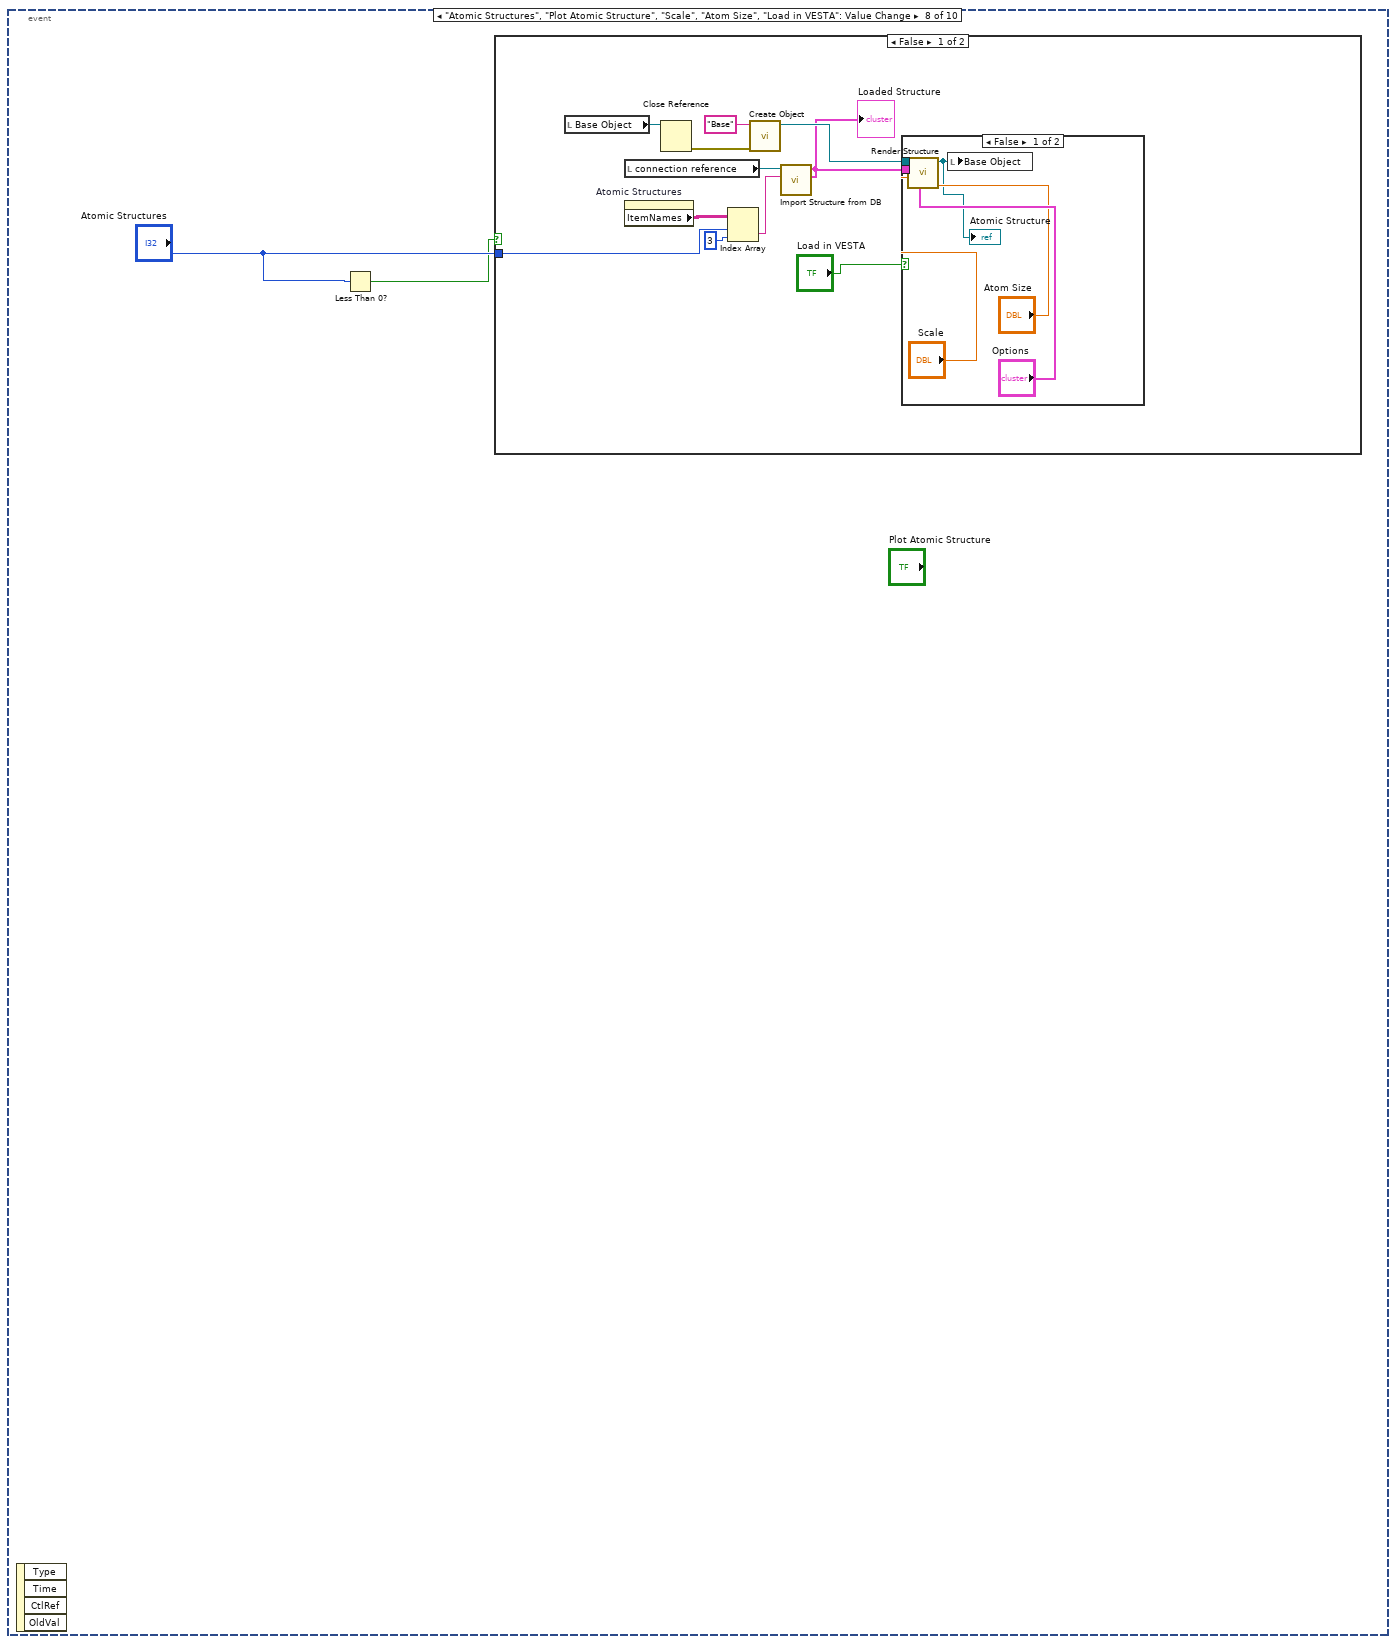
[diagram p19: hidden frame]
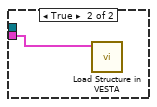
[diagram p20: hidden frame]
diagram:
  n1 = call-poly <vilib>:"DB Tools Open Connection.vi"("connection information"="UDL") -> ("error out"=w6:errorcluster, "connection reference"=w14:T6)  [unwired: 7 in]
  n2 = call-poly <vilib>:"DB Tools Execute Query.vi"("error in (no error)"=w6, "SQL query"="SELECT DISTINCT [0D_Point_Defects].Defect_Free_Structure_ID, [0D_Point_Defects].Defect_Free_Structure_Name, [0D_Point_Defects].[Defect_Free_Energy_(eV)]\nFROM [0D_Point_Defects];\n", "connection reference"=w14) -> ("error out"=w16:errorcluster, "recordset reference"=w13:T9)  [unwired: 5 in]
  n3 = call "Column Headers from SQL Query Recordset.vi"("error in (no error)"=w16, "recordset reference"=w13) -> ("error out"=w15:errorcluster, "columns"=w7:string[], "Recordset reference Out"=w12:T9)  [unwired: 6 in, 1 out]
  n4 = call-poly <vilib>:"DB Tools Fetch Recordset Data.vi"("error in (no error)"=w15, "recordset reference"=w12) -> ("error out"=w17:errorcluster, "recordset data"=w9:variant[][], "recordset reference out"=w11:T9)  [unwired: 3 in]
  n5 = for {
    tunnel: w9 -> [w20] mode=indexing
    tunnel: [w19] -> w8 mode=indexing
    n6 = for {
      tunnel: w20 -> [w23] mode=indexing
      tunnel: [w21] -> w19 mode=indexing
      n7 = xnode "Database Variant To Data"("database variant"=w23, "type"="") -> ("data"=w21:string)  [unwired: 1 in, 1 out]
    }
  }
  n8 = call-poly <vilib>:"DB Tools Free Object.vi"("error in (no error)"=w17, "recordset reference"=w11) -> ("connection reference"=w1:T6)  [unwired: 8 in, 1 out]
  "connection reference" <- w1
  n9 = call <vilib>:"Create Object.vi"("Name"="Base") -> ("error out"=w2:errorcluster, "Scene:New Object"=→"Base Object":refnum<vi>)  [unwired: 1 in, 8 out]
  n10 = property on="Pure Structures with defects" class="MCListbox (strict)"(error in=w2, "ColHdrString"=w7, "ItemNames"=w8) -> (error out=w5:errorcluster)  [unwired: 1 in, 1 out]
  n11 = while {
    tunnel: w5 -> [_]
    tunnel: w1 -> [_]
    stop <- FALSE stop-if-true
    n12 = event shown="[6] \"Bound Pairs List\": Value Change" {
      selector: _ -> [_ _ _ _ _ _ _ _ _ _]
      dyn-events: _ -> [_ _ _ _ _ _ _ _ _ _]
      timeout: 60000 -> [_ _ _ _ _ _ _ _ _ _]
      event Timeout {
        n13 = event-data() -> ()  [unwired: 1 in, 2 out]
        n14 = Wait (ms)(milliseconds to wait=u32 10) -> ()  [unwired: 1 out]
      }
      event "Pure Structures with defects", "Chemical Potential", "Chemical Potential 2", "Thermodynamic Fermi Level": Value Change {
        w73 = -1.0 ("Thermodynamic Fermi Level (eV)")
        w79 = T11 {"Name"="Thermodynamic Fermi Level", "Color"=0, "Style"=2, "Point Style"=13, "Name Visible"=TRUE, "Allow Drag"=TRUE, "Cursor Mode"=0, "Plot"=0, "Index"=0, "Position"={"X"=2.4701149425287356, "Y"=0.0}, "X Scale"=0, "Y Scale"=0, "Watch Plots"=[], "Watch All Plots"=FALSE, "Plot Area"=0, "Label Offset"={"X"=0.016091954022988464, "Y"=2.3061224489795915}} ("element")
        n15 = event-data() -> ()  [unwired: 1 in, 3 out]
        n16 = property on="Pure Structures with defects" class="MCListbox (strict)"() -> ("ItemNames"=w88:string[][])  [unwired: 2 in, 2 out]
        n17 = local read "connection reference"() -> (w84:T6)
        n18 = Index Array(array=w88, index (col) #1=0 ("disabled index (col)")) -> (element #1=w85:string[], element #2=w67:string[])  [unwired: 3 in]
        n19 = for {
          tunnel: "Pure Structures with defects" -> [w90] mode=indexing
          tunnel: w85 -> [w122]
          shift-right: [w120] -> _
          shift-left: w84 -> [w121]
          shift-right: [w111] -> w62
          shift-left: string[][] [] -> [w110]
          tunnel: "Calc Thermodynamic Fermi Level" -> [w109]
          shift-right: [w116] -> w72
          shift-left: w73 -> [w106]
          shift-right: [w117] -> w71
          shift-left: w73 -> [w105]
          tunnel: [w103] -> w70 mode=indexing
          shift-right: [w99] -> w68
          shift-left: cluster{i32, i32}[] [] -> [w98]
          tunnel: w67 -> [w97]
          tunnel: dbl[] [5230.5515143, 4360.60278, 2309.371815, 7792.576126] ("Volumes 2") -> [w92]
          tunnel: [w91] -> w59 mode=indexing
          i -> [w101]
          n20 = Index Array(array=w122, index=w90) -> (element=w104:string)
          n21 = Index Array(array=w97, index=w90) -> (element=w96:string)
          n22 = Index Array(array=w92, index=w90) -> (element=w91:dbl)
          n23 = property on="Pure Structures with defects" class="MCListbox (strict)"() -> ("ItemNames"=w115:string[][])  [unwired: 2 in, 2 out]
          n24 = local read "Chemical Potential 2"() -> (w118:dbl)
          n25 = local read "Chemical Potential"() -> (w119:dbl)
          n26 = Equal?(x="Thermodynamic Fermi Level", y=w90) -> (x = y?=w108:bool)
          n27 = call "DB Get Defects from pure ID.vi"("Ignore Location"="Ignore Location", "Defect Free Structure ID"=w104, "connection reference in"=w121) -> ("Defects Array"=w102:T12, "connection reference out"=w120:T6)  [unwired: 5 in, 2 out]
          n28 = Index Array(array=w115, index (row)=w90, index (col)=1 ("disabled index (col)")) -> (element=w113:string)
          n29 = Index Array(array=w92, index="Thermodynamic Fermi Level") -> (element=w93:dbl)
          n30 = for {
            tunnel: [w136] -> w112 mode=indexing
            tunnel: w113 -> [w135]
            tunnel: w102 -> [w134] mode=indexing
            tunnel: w101 -> [w132]
            tunnel: [w131] -> w100 mode=indexing
            i -> [w133]
            n31 = Unbundle By Name(w134) -> ("Defect Details"=w139:T13, "Charges and Energies"=w141:T14)
            n32 = Unbundle By Name(w139) -> ("Defect Name"=w138:string)
            n33 = for {
              tunnel: w141 -> [w147] mode=indexing
              shift-right: [w146] -> w137
              shift-left: "" -> [w145]
              n34 = Unbundle By Name(w147) -> ("Net Charge"=w144:i32)
              n35 = Number To Decimal String(number=w144) -> (decimal integer string=w143:string)  [unwired: 1 in]
              n36 = Concatenate Strings(w145, w143, ", " ("string")) -> (w146:string)
            }
            n37 = Build Array(w135, w138, w137) -> (w136:string[])
            n38 = Bundle(w132, w133) -> (w131:cluster{i32, i32})  [unwired: 1 in]
          }
          n39 = And(x=w109, y=w108) -> (x .and. y?=w107:bool)
          n40 = case shown="True" w107 {
            tunnel: w119 -> [_ w130]
            tunnel: w118 -> [_ w129]
            tunnel: [w123 w128] -> w117
            tunnel: [w124 w127] -> w116
            tunnel: w102 -> [_ w126]
            tunnel: w106 -> [w124 _]
            tunnel: w105 -> [w123 _]
            tunnel: w93 -> [_ w125]
            frame False {
            }
            frame True {
              n41 = call "Self-consistent charge neutrality.vi"("Volume (A³)"=w125, "Chemical Potential (0=Cd, 1=Te)"=w129, "Defects"=w126) -> ("Thermodynamic Fermi Level (eV) - VBM"=w127:dbl)  [unwired: 8 in]
              n42 = call "Self-consistent charge neutrality.vi"("Volume (A³)"=w125, "Chemical Potential (0=Cd, 1=Te)"=w130, "Defects"=w126) -> ("Thermodynamic Fermi Level (eV) - VBM"=w128:dbl)  [unwired: 8 in]
            }
          }
          n43 = Bundle(w96, "Defects Array"=w102) -> (w103:T15)  [unwired: 1 in]
          n44 = Build Array (concatenate)(w110, w112) -> (w111:string[][])
          n45 = Build Array (concatenate)(w98, w100) -> (w99:cluster{i32, i32}[])
        }
        "Thermodynamic Fermi Level (eV)" <- w71
        "All Hosts and Defects" <- w70
        "Indicies" <- w68
        "Array" <- w62
        n46 = Array To Spreadsheet String(delimiter (Tab)=",", array=w62, 3:"\\s" ("format string")) -> (spreadsheet string=→"spreadsheet string":string)
        n47 = disable-structure shown="Enabled" {
          disable-tunnel: [_ w89] -> w78
          frame Disabled {
          }
          frame Enabled {
            n48 = local read "Related Defects"() -> (w89:i32[])
          }
        }
        n49 = Index Array(array=w62, index (col)=1 ("disabled index (col)")) -> (element=w66:string[])  [unwired: 1 in]
        n50 = property on="Related Defects" class="MCListbox (strict)"("ColHdrString"=string[] ["Defect Free Structure", "Defect Name", "Net Charges"] ("Column Header Strings[]"), "ItemNames"=w62) -> (error out=w75:errorcluster)  [unwired: 2 in, 1 out]
        n51 = local write "Volumes"(w59) -> ()
        n52 = Bundle By Name(cluster=w79, "Position.X"=w72) -> (w80:T11)
        n53 = Bundle By Name(cluster=w79, "Position.X"=w71) -> (w82:T11)
        n54 = property on="Related Defects" class="MCListbox (strict)"(error in=w75, "Val(Sgnl)"=w78) -> ()  [unwired: 1 in, 2 out]
        n55 = Build Array(w80) -> (w81:T16)
        n56 = Build Array(w82) -> (w83:T16)
        n57 = property on="Defect" class="CmbBox"("Strings[]"=w66) -> ()  [unwired: 2 in, 2 out]
        n58 = property on="Te Rich Limit" class="XYGraph (strict)"("CrsrList"=w81) -> ()  [unwired: 2 in, 2 out]
        n59 = property on="Cd Rich Limit" class="XYGraph (strict)"("CrsrList"=w83) -> ()  [unwired: 2 in, 2 out]
      }
      event "Related Defects", "Show Charge Transitions", "Markov-Payne Correction": Value Change {
        w164 = T17 []
        n60 = event-data() -> ()  [unwired: 1 in, 4 out]
        n61 = local read "All Hosts and Defects"() -> (w154:T4)
        n62 = for {
          N -> [w203]
          tunnel: w154 -> [w189]
          tunnel: [w209] -> w159 mode=indexing
          tunnel: [w207] -> w161 mode=indexing
          tunnel: [w182] -> w151 mode=indexing
          tunnel: [w203] -> w168
          tunnel: "Related Defects" -> [w191] mode=indexing
          shift-right: [w197] -> w163
          shift-left: w164 -> [w201]
          tunnel: T10 {"Name"="0 / +1", "Color"=0, "Style"=4, "Point Style"=1, "Name Visible"=TRUE, "Allow Drag"=TRUE, "Annotation Mode"=0, "Plot"=-1, "Index"=0, "Position"={"X"=2.0, "Y"=1.0}, "X Scale"=0, "Y Scale"=0, "Show Arrow"=FALSE, "Lock Name"=FALSE, "Plot Area"=0, "Label Offset"={"X"=0.0, "Y"=0.05}} ("element 2") -> [w200]
          shift-right: [w196] -> w162
          shift-left: w164 -> [w198]
          tunnel: [w193] -> w156 mode=indexing
          shift-right: [w180] -> w152
          shift-left: string[][] [] -> [w179]
          n63 = local read "Indicies"() -> (w192:cluster{i32, i32}[])
          n64 = Index Array(array=w192, index=w191) -> (element=w190:cluster{i32, i32})
          "element 2" <- w190
          n65 = local read "VBM"() -> (w175:dbl)
          n66 = call "Start and End to Array 2.vi"("Sweep Style"=enum16{"Linear Step", "Linear Pts", "Log Pts"}."Linear Pts", "Step or # Pts"=100.0, "End"=3.4, "Start"=w175) -> ("Array"=w199:dbl[])  [unwired: 7 in]
          n67 = Unbundle(w190) -> (w178:i32, w186:i32)
          n68 = Index Array(array="Volumes", index=w178) -> (element=w176:dbl)
          n69 = Index Array(array=w189, index=w178) -> (element=w188:T18)
          n70 = Build Array (concatenate)(w199) -> (w195:dbl[])
          n71 = Unbundle(w188) -> ("Defect Free Name"=w183:string, "Defects Array"=w187:T12)
          n72 = Index Array(array=w187, index=w186) -> (element=w185:T19)
          n73 = Unbundle By Name(w185) -> ("Defect Details.Defect Name"=w182:string, "Charges and Energies"=w184:T14)
          n74 = case shown="True" "Show Charge Transitions" {
            tunnel: w185 -> [_ w232]
            tunnel: w201 -> [_ w230]
            tunnel: w200 -> [_ w231]
            tunnel: w198 -> [_ w227]
            tunnel: [_ w228] -> w197
            tunnel: [_ w225] -> w196
            tunnel: w182 -> [_ w223]
            tunnel: [_ w222] -> w193
            tunnel: w176 -> [_ w221]
            frame False {
            }
            frame True {
              n75 = local read "VBM"() -> (w219:dbl)
              n76 = local read "Markov-Payne Correction"() -> (w220:bool)
              n77 = call "Find Charge Transitions.vi"("Dielectric Constant"=11.0, "Volume (A³)"=w221, "Markov-Payne Corrections"=w220, "VBM"=w219, "Defect Data"=w232) -> ("Transitions"=w224:T20)  [unwired: 6 in]
              n78 = for {
                tunnel: w224 -> [w247] mode=indexing
                tunnel: w231 -> [w245]
                tunnel: [w241] -> w229 mode=indexing
                tunnel: [w240] -> w226 mode=indexing
                n79 = local read "Chemical Potential 2"() -> (w234:dbl)
                n80 = local read "Chemical Potential"() -> (w237:dbl)
                n81 = Unbundle(w247) -> ("Transition"=w244:string, "Fermi Energy (eV)"=w243:dbl, "Formation Energy, Cd Rich (eV)"=w239:dbl, "Formation Energy, Te Rich (eV)"=w238:dbl)
                n82 = Build Array(w239, w238) -> (w235:dbl[])
                n83 = Interpolate 1D Array(1:w237, 2:w235) -> (0:w236:dbl)
                n84 = Interpolate 1D Array(1:w234, 2:w235) -> (0:w233:dbl)
                n85 = Bundle("Fermi Energy (eV)"=w243, w236) -> (w246:cluster{"Fermi Energy (eV)":dbl, dbl})  [unwired: 1 in]
                n86 = Bundle("Fermi Energy (eV)"=w243, w233) -> (w242:cluster{"Fermi Energy (eV)":dbl, dbl})  [unwired: 1 in]
                n87 = Bundle By Name(cluster=w245, "Name"=w244, "Position"=w246) -> (w241:T10)
                n88 = Bundle By Name(cluster=w245, "Name"=w244, "Position"=w242) -> (w240:T10)
              }
              n89 = Bundle("Defect Name"=w223, "Transitions"=w224) -> (w222:T21)  [unwired: 1 in]
              n90 = Build Array (concatenate)(w230, w229) -> (w228:T17)
              n91 = Build Array (concatenate)(w227, w226) -> (w225:T17)
            }
          }
          n92 = for {
            tunnel: w195 -> [w254] mode=indexing
            tunnel: [w253] -> w210 mode=indexing
            tunnel: [w252] -> w208 mode=indexing
            tunnel: w185 -> [w251]
            tunnel: w176 -> [w249]
            w248 = 11.0 ("Dielectric Constant")
            n93 = call "Calc Formation Energy from Defect Cluster.vi"("Dielectric Constant"=w248, "Volume (A³)"=w249, "Markov-Payne Correction"="Markov-Payne Correction", "Chemical Potential"="Chemical Potential 2", "Fermi Level (eV)"=w254, "Defect Data"=w251) -> ("Formation Energy (eV)"=w252:dbl)  [unwired: 4 in, 1 out]
            n94 = call "Calc Formation Energy from Defect Cluster.vi"("Dielectric Constant"=w248, "Volume (A³)"=w249, "Markov-Payne Correction"="Markov-Payne Correction", "Chemical Potential"="Chemical Potential", "Fermi Level (eV)"=w254, "Defect Data"=w251) -> ("Formation Energy (eV)"=w253:dbl)  [unwired: 4 in, 1 out]
          }
          n95 = for {
            tunnel: w184 -> [w217] mode=indexing
            tunnel: w183 -> [w214]
            tunnel: w182 -> [w213]
            tunnel: [w212] -> w181 mode=indexing
            n96 = Unbundle By Name(w217) -> ("Net Charge"=w216:i32, "Structure ID"=w211:string)
            n97 = Number To Decimal String(number=w216) -> (decimal integer string=w215:string)  [unwired: 1 in]
            n98 = Build Array(w214, w213, w215, w211) -> (w212:string[])
          }
          n99 = Build Array (concatenate)(w179, w181) -> (w180:string[][])
          n100 = Subtract(x=w195, y=w175) -> (x-y=w194:dbl[])
          n101 = Bundle(w194, w208) -> (w207:cluster{dbl[], dbl[]})  [unwired: 1 in]
          n102 = Bundle(w194, w210) -> (w209:cluster{dbl[], dbl[]})  [unwired: 1 in]
        }
        "Cd Rich Limit" <- w159
        "Te Rich Limit" <- w161
        "Array 2" <- w156
        n103 = local read "Plots Tab"() -> (w160:T7)
        n104 = case shown="\"Binding Energy\"" w160 {
          frame "Formation Energies vs Fermi", Default {
          }
          frame "Binding Energy" {
            n105 = property on="Plot Binding Energy" class="Bool (strict)"("Val(Sgnl)"=TRUE ("Value (Signaling)")) -> ()  [unwired: 2 in, 2 out]
          }
          frame "Charge Transition Levels" {
          }
          frame "Atomic Structure" {
          }
        }
        n106 = property on="Atomic Structures" class="MCListbox (strict)"("ItemNames"=w152) -> ()  [unwired: 2 in, 2 out]
        n107 = property on="Te Rich Limit" class="XYGraph (strict)"("AnntList"=w162) -> ()  [unwired: 2 in, 2 out]
        n108 = property on="Cd Rich Limit" class="XYGraph (strict)"("AnntList"=w163) -> ()  [unwired: 2 in, 2 out]
        n109 = control-ref of="Defect Energy Levels"() -> (w157:refnum<vi>)
        n110 = disable-structure shown="Enabled" {
          disable-tunnel: w156 -> [w170 w173]
          disable-tunnel: [w169 w173] -> w155
          frame Disabled {
            n111 = Decimate 1D Array(w170) -> (w172:T2, w171:T2)
            n112 = Build Array (concatenate)(w172, w171) -> (w169:T2)
          }
          frame Enabled {
          }
        }
        n113 = call "Make Defect Energy Transition Plot.vi"("Buckets"="Buckets", "All Defects and Transitions"=w155, "XY Graph Reference"=w157) -> ()  [unwired: 9 in]
        n114 = call "Num of Colors to Color Array.vi"("# of Colors"=w168, "Color Array Type"="Color Array Type") -> ("Colors Array"=w149:u32[])  [unwired: 3 in]
        n115 = control-ref of="Te Rich Limit"() -> (w158:refnum<vi>)
        n116 = control-ref of="Cd Rich Limit"() -> (w167:refnum<vi>)
        n117 = call "Format XY Plot.vi"("Colors Array"=w149, "Plot Names"=w151, "XY Graph Reference"=w158) -> ()  [unwired: 9 in]
        n118 = call "Format XY Plot.vi"("Colors Array"=w149, "Plot Names"=w151, "XY Graph Reference"=w167) -> ()  [unwired: 9 in]
      }
      event "Save as a table": Value Change {
        n119 = event-data() -> ()  [unwired: 1 in, 4 out]
        n120 = call "Fermi Level?"() -> ("Fermi Level"=w257:dbl, "OK"=w258:bool)  [unwired: 17 in, 1 out]
        n121 = case shown="True" w258 {
          tunnel: w257 -> [_ w266]
          frame False {
          }
          frame True {
            n122 = Less Or Equal To 0?(x=w266) -> (x <= 0?=w267:bool)
            n123 = local read "All Hosts and Defects"() -> (w259:T4)
            n124 = local read "Related Defects"() -> (w283:i32[])
            n125 = case shown="False" w267 {
              tunnel: [w284 w285] -> w260
              tunnel: w266 -> [w284 _]
              frame False {
              }
              frame True {
                n126 = local read "Thermodynamic Fermi Level (eV)"() -> (w285:dbl)
              }
            }
            n127 = Add(x="VBM", y=w260) -> (x+y=w272:dbl)
            n128 = for {
              tunnel: w283 -> [w293] mode=indexing
              tunnel: [w304] -> w282 mode=indexing
              tunnel: [w303] -> w281 mode=indexing
              tunnel: w272 -> [w302]
              tunnel: [w301] -> w265 mode=indexing
              tunnel: [w299] -> w263 mode=indexing
              tunnel: w259 -> [w294]
              n129 = local read "Indicies"() -> (w298:cluster{i32, i32}[])
              n130 = Index Array(array=w298, index=w293) -> (element=w297:cluster{i32, i32})
              "element" <- w297
              n131 = Unbundle(w297) -> (w288:i32, w295:i32)
              n132 = local read "Markov-Payne Correction"() -> (w290:bool)
              n133 = local read "Chemical Potential"() -> (w305:dbl)
              n134 = Index Array(array=w294, index=w288) -> (element=w296:T18)
              n135 = local read "Volumes"() -> (w289:dbl[])
              n136 = Index Array(array=w289, index=w288) -> (element=w287:dbl)
              n137 = Unbundle(w296) -> ("Defects Array"=w292:T12)  [unwired: 1 out]
              n138 = Index Array(array=w292, index=w295) -> (element=w291:T19)
              n139 = call "Calc Formation Energy from Defect Cluster.vi"("Dielectric Constant"=11.0, "Volume (A³)"=w287, "Markov-Payne Correction"=w290, "Chemical Potential"=w305, "Fermi Level (eV)"=w302, "Defect Data"=w291) -> ("Net Charge"=w301:i32, "Formation Energy (eV)"=w304:dbl)  [unwired: 4 in]
              n140 = Unbundle By Name(w291) -> ("Defect Details.Defect Name"=w303:string, "Defect Details.Reference Pure Structure Energy"=w300:dbl)
              n141 = Number To Fractional String(number=w300) -> (F-format string=w299:string)  [unwired: 3 in]
            }
            n142 = Number To Fractional String(number="VBM") -> (F-format string=w261:string)  [unwired: 3 in]
            n143 = local read "Chemical Potential"() -> (w277:dbl)
            n144 = Number To Fractional String(number=w277) -> (F-format string=w276:string)  [unwired: 3 in]
            n145 = Number To Fractional String(number=w260) -> (F-format string=w278:string)  [unwired: 3 in]
            n146 = Number To Fractional String(number=w282) -> (F-format string=w280:string[])  [unwired: 3 in]
            n147 = Number To Decimal String(number=w265) -> (decimal integer string=w264:string[])  [unwired: 1 in]
            n148 = Build Array(w276, w278, w261) -> (w274:string[])
            n149 = Build Array(w281, w263, w280, w264) -> (w279:string[][])
            n150 = Build Array(string[] ["Chemical Potential (% Te Rich)", "Fermi Energy (eV)", "VBM"], w274) -> (w273:string[][])
            n151 = Transpose 2D Array(2D array=w279) -> (transposed array=w269:string[][])
            n152 = Build Array (concatenate)(w273, string[] [" "] ("element"), string[] ["Defect Name", "Defect Free Energy", "Formation Energy (eV)", "Net Charge"], w269) -> (w271:string[][])
            n153 = call-poly <vilib>:"Write To Spreadsheet File.vi"("2D data"=w271) -> ()  [unwired: 7 in, 1 out]
          }
        }
      }
      event "Set as seperate defects": Value Change {
        n154 = event-data() -> ()  [unwired: 1 in, 4 out]
        n155 = local read "Related Defects"() -> (w308:i32[])
        n156 = local read "Indicies"() -> (w307:cluster{i32, i32}[])
        n157 = for {
          tunnel: w308 -> [w313] mode=indexing
          tunnel: w307 -> [w314]
          tunnel: [w312] -> w306 mode=indexing
          n158 = Index Array(array=w314, index=w313) -> (element=w312:cluster{i32, i32})
        }
        "Separate Defects" <- w306
        n159 = property on="Related Defects" class="MCListbox (strict)"() -> ("Value"=w311:i32[], "ItemNames"=w310:string[][])  [unwired: 2 in, 2 out]
        n160 = for {
          tunnel: w311 -> [w318] mode=indexing
          tunnel: w310 -> [w317]
          tunnel: [w315] -> w309 mode=indexing
          n161 = Index Array(array=w317, index (row)=w318, index (col)=1 ("disabled index (col)")) -> (element=w315:string)
        }
        n162 = property on="Seperate Defects" class="LstBox (strict)"("Item Names"=w309) -> ()  [unwired: 2 in, 2 out]
      }
      event "Assign Bound Calculation": Value Change {
        n163 = event-data() -> ()  [unwired: 1 in, 4 out]
        n164 = property on="Related Defects" class="MCListbox (strict)"() -> ("Value"=w323:i32[], "ItemNames"=w325:string[][])  [unwired: 2 in, 2 out]
        n165 = local read "Related Defects"() -> (w333:i32[])
        n166 = Index Array(array=w323) -> (element=w322:i32)  [unwired: 1 in]
        n167 = local read "Separate Defects"() -> (w329:cluster{i32, i32}[])
        n168 = local read "Indicies"() -> (w332:cluster{i32, i32}[])
        n169 = property on="Bound Pairs List" class="LstBox (strict)"() -> ("Item Names"=w321:string[])  [unwired: 2 in, 2 out]
        n170 = Index Array(array=w333) -> (element=w331:i32)  [unwired: 1 in]
        n171 = Index Array(array=w325, index (row)=w322, index (col)=1 ("disabled index (col)")) -> (element=w319:string)
        n172 = Index Array(array=w332, index=w331) -> (element=w330:cluster{i32, i32})
        n173 = Build Array (concatenate)(w321, w319) -> (w320:string[])
        n174 = Bundle(w330, "Separate Defects"=w329) -> (w327:T22)  [unwired: 1 in]
        n175 = property on="Bound Pairs List" class="LstBox (strict)"("Item Names"=w320) -> ()  [unwired: 2 in, 2 out]
        n176 = Build Array (concatenate)("Bound Pairs", w327) -> (w326:T1)
        n177 = local write "Bound Pairs"(w326) -> ()
      }
      event "Bound Pairs List": Value Change {
        n178 = event-data() -> ()  [unwired: 1 in, 4 out]
        n179 = local read "Markov-Payne Correction"() -> (w334:bool)
        n180 = local read "All Hosts and Defects"() -> (w335:T4)
        n181 = local read "VBM"() -> (w337:dbl)
        n182 = local read "Defects to Bind"() -> (w372:i32[])
        n183 = local read "Bound Pairs"() -> (w340:T1)
        n184 = call "Start and End to Array 2.vi"("Sweep Style"=enum16{"Linear Step", "Linear Pts", "Log Pts"}."Linear Pts", "Step or # Pts"=30.0, "End"=3.4, "Start"=w337) -> ("Array"=w338:dbl[])  [unwired: 7 in]
        n185 = Subtract(x=w338, y=w337) -> (x-y=w336:dbl[])
        n186 = for {
          tunnel: "Bound Pairs List" -> [w380] mode=indexing
          tunnel: w340 -> [w381]
          tunnel: w338 -> [w377]
          tunnel: "Binding Energy Chem Pot" -> [w376]
          tunnel: w336 -> [w373]
          tunnel: w335 -> [w375]
          tunnel: w334 -> [w374]
          n187 = Index Array(array=w381, index=w380) -> (element=w379:T23)
          n188 = Unbundle(w379) -> ("Separate Defects"=w378:T24)  [unwired: 1 out]
          n189 = for {
            tunnel: w378 -> [w392] mode=indexing
            tunnel: w377 -> [w387]
            tunnel: w376 -> [w386]
            tunnel: w375 -> [w393]
            tunnel: w374 -> [w385]
            n190 = Unbundle(w392) -> ("Host Crystal Index"=w383:i32, "Defect Index"=w389:i32)
            n191 = local read "Volumes"() -> (w384:dbl[])
            n192 = Index Array(array=w393, index=w383) -> (element=w391:T18)
            n193 = Unbundle(w391) -> ("Defects Array"=w390:T12)  [unwired: 1 out]
            n194 = Index Array(array=w384, index=w383) -> (element=w382:dbl)
            n195 = Index Array(array=w390, index=w389) -> (element=w388:T19)
            n196 = for {
              tunnel: w388 -> [w400]
              tunnel: w387 -> [w399] mode=indexing
              tunnel: w386 -> [w398]
              tunnel: w385 -> [w397]
              tunnel: [w396] -> _ mode=indexing
              tunnel: w382 -> [w394]
              n197 = call "Calc Formation Energy from Defect Cluster.vi"("Dielectric Constant"=11.0, "Volume (A³)"=w394, "Markov-Payne Correction"=w397, "Chemical Potential"=w398, "Fermi Level (eV)"=w399, "Defect Data"=w400) -> ("Formation Energy (eV)"=w396:dbl)  [unwired: 4 in, 1 out]
            }
          }
          n198 = Bundle(w373) -> ()  [unwired: 2 in, 1 out]
        }
        n199 = for {
          N -> [w431]
          tunnel: [w431] -> _
          tunnel: w372 -> [w429] mode=indexing
          tunnel: w338 -> [w430]
          tunnel: [w427] -> w366 mode=indexing
          tunnel: "Binding Energy Chem Pot" -> [w426]
          tunnel: w335 -> [w425]
          n200 = for {
            tunnel: w430 -> [w446] mode=indexing
            tunnel: [w444] -> w428 mode=indexing
            tunnel: w429 -> [w437]
            tunnel: w426 -> [w445]
            tunnel: w425 -> [w438]
            n201 = local read "Markov-Payne Correction"() -> (w435:bool)
            n202 = local read "Indicies"() -> (w439:cluster{i32, i32}[])
            n203 = local read "Volumes"() -> (w434:dbl[])
            n204 = Index Array(array=w439, index=w437) -> (element=w440:cluster{i32, i32})
            n205 = Unbundle(w440) -> (w433:i32, w442:i32)
            n206 = Index Array(array=w434, index=w433) -> (element=w432:dbl)
            n207 = Index Array(array=w438, index=w433) -> (element=w441:T18)
            n208 = Unbundle(w441) -> ("Defects Array"=w443:T12)  [unwired: 1 out]
            n209 = Index Array(array=w443, index=w442) -> (element=w436:T19)
            n210 = call "Calc Formation Energy from Defect Cluster.vi"("Volume (A³)"=w432, "Markov-Payne Correction"=w435, "Chemical Potential"=w445, "Fermi Level (eV)"=w446, "Defect Data"=w436) -> ("Formation Energy (eV)"=w444:dbl)  [unwired: 5 in, 1 out]
          }
          n211 = Add Array Elements(numeric array=w428) -> (sum=w427:dbl)
        }
        n212 = local read "Related Defects"() -> (w368:i32[])
        n213 = Subtract(x=w338, y=w337) -> (x-y=w359:dbl[])
        n214 = Bundle(w359, w366) -> (w367:cluster{dbl[], dbl[]})  [unwired: 1 in]
        n215 = for {
          tunnel: w368 -> [w402] mode=indexing
          tunnel: [w420] -> w364 mode=indexing
          tunnel: w359 -> [w419]
          tunnel: [w418] -> w363 mode=indexing
          tunnel: w366 -> [w416]
          tunnel: "Binding Energy Chem Pot" -> [w414]
          tunnel: [w412] -> w361 mode=indexing
          tunnel: [w411] -> w353 mode=indexing
          tunnel: w338 -> [w410]
          tunnel: w335 -> [w403]
          n216 = local read "Indicies"() -> (w404:cluster{i32, i32}[])
          n217 = Index Array(array=w404, index=w402) -> (element=w405:cluster{i32, i32})
          n218 = Unbundle(w405) -> (w406:i32, w408:i32)
          n219 = Index Array(array=w403, index=w406) -> (element=w407:T18)
          n220 = Unbundle(w407) -> ("Defects Array"=w409:T12)  [unwired: 1 out]
          n221 = Index Array(array=w409, index=w408) -> (element=w401:T19)
          n222 = Unbundle By Name(w401) -> ("Defect Details.Defect Name"=w411:string)
          n223 = for {
            tunnel: w410 -> [w424] mode=indexing
            tunnel: [w423] -> w417 mode=indexing
            tunnel: w414 -> [w422]
            tunnel: w401 -> [w421]
            n224 = call "Calc Formation Energy from Defect Cluster.vi"("Chemical Potential"=w422, "Fermi Level (eV)"=w424, "Defect Data"=w421) -> ("Formation Energy (eV)"=w423:dbl)  [unwired: 7 in, 1 out]
          }
          n225 = Subtract(x=w417, y=w416) -> (x-y=w415:dbl[])
          n226 = Concatenate Strings("Binding of " ("string"), w411) -> (w412:string)
          n227 = Bundle(w419, w415) -> (w418:cluster{dbl[], dbl[]})  [unwired: 1 in]
          n228 = Bundle(w419, w417) -> (w420:cluster{dbl[], dbl[]})  [unwired: 1 in]
        }
        n229 = local read "Color Array Type"() -> (w356:T5)
        n230 = Interleave 1D Arrays(w364, w363) -> (w362:cluster{dbl[], dbl[]}[])
        n231 = Interleave 1D Arrays(w353, w361) -> (w357:string[])
        n232 = Array Size(array=w353) -> (size(s)=w347:i32)
        n233 = Build Array (concatenate)(w367, w362) -> (→"Binding Energy":cluster{dbl[], dbl[]}[])
        n234 = call "Num of Colors to Color Array.vi"("# of Colors"=w347, "Color Array Type"=w356) -> ("Colors Array"=w352:u32[])  [unwired: 3 in]
        n235 = Initialize Array(0, w347) -> (w345:i32[])
        n236 = Initialize Array(1, w347) -> (w344:i32[])
        n237 = Build Array (concatenate)("Seperate" ("String"), w357) -> (w358:string[])
        n238 = Interleave 1D Arrays(w352, w352) -> (w351:u32[])
        n239 = Interleave 1D Arrays(w345, w344) -> (w343:i32[])
        n240 = control-ref of="Binding Energy"() -> (w350:refnum<vi>)
        n241 = Build Array (concatenate)(0, w343) -> (w342:i32[])
        n242 = Build Array (concatenate)(u32 0 ("Color Box"), w351) -> (w354:u32[])
        n243 = call "Format XY Plot.vi"("Active Y Scale (Left or Right)"=w342, "Line Styles"=w342, "Colors Array"=w354, "Plot Names"=w358, "XY Graph Reference"=w350) -> ()  [unwired: 7 in]
      }
      event "Atomic Structures", "Plot Atomic Structure", "Scale", "Atom Size", "Load in VESTA": Value Change {
        n244 = event-data() -> ()  [unwired: 1 in, 4 out]
        n245 = Less Than 0?(x="Atomic Structures") -> (x < 0?=w447:bool)
        n246 = case shown="False" w447 {
          tunnel: "Atomic Structures" -> [w451 _]
          frame False {
            n247 = local read "Base Object"() -> (w457:refnum<vi>)
            n248 = local read "connection reference"() -> (w452:T6)
            n249 = property on="Atomic Structures" class="MCListbox (strict)"() -> ("ItemNames"=w455:string[][])  [unwired: 2 in, 2 out]
            n250 = Close Reference(reference=w457) -> (error out=w456:errorcluster)  [unwired: 1 in]
            n251 = Index Array(array=w455, index (row)=w451, index (col)=3 ("disabled index (col)")) -> (element=w453:string)
            n252 = call <vilib>:"Create Object.vi"("error in (no error)"=w456, "Name"="Base") -> ("Scene:New Object"=w458:refnum<vi>)  [unwired: 9 out]
            n253 = call "Import Structure from DB.vi"("Structure ID"=w453, "connection reference"=w452) -> ("Loaded Structure"=w450:T3)  [unwired: 7 in, 2 out]
            "Loaded Structure" <- w450
            n254 = case shown="False" "Load in VESTA" {
              tunnel: w458 -> [w463 _]
              tunnel: w450 -> [w461 w466]
              frame False {
                n255 = call "Render Structure.vi"("Options"="Options", "Atom Size"="Atom Size", "Scale"="Scale", "Atomic Structure"=w461, "Base Object"=w463) -> ("Object with atoms"=w460:refnum<vi>)  [unwired: 6 in]
                "Atomic Structure" <- w460
                n256 = local write "Base Object"(w460) -> ()
              }
              frame True {
                n257 = call "Load Structure in VESTA.vi"("Atomic Structure"=w466) -> ()  [unwired: 11 in]
              }
            }
          }
          frame True {
          }
        }
      }
      event "Setup Camera": Value Change {
        n258 = event-data() -> ()  [unwired: 1 in, 4 out]
        n259 = local read "Loaded Structure"() -> (w482:T3)
        n260 = control-ref of="Atomic Structure"() -> (w467:refnum<vi>)
        n261 = Unbundle By Name(w482) -> ("Lattice vector a"=w472:dbl[], "Lattice vector b"=w471:dbl[], "Lattice vector c"=w481:dbl[])
        n262 = Negate(x=w472) -> (-x=w470:dbl[])
        n263 = Compound Arithmetic op=ADD(w472, w471, w481) -> (w479:dbl[])
        n264 = local read "Scale"() -> (w478:dbl)
        n265 = Divide(x=w479, y=2.0) -> (x/y=w477:dbl[])
        n266 = Multiply(x=w477, y=w478) -> (x*y=w476:dbl[])
        n267 = Multiply(x=w470, y=2.0 ("Numeric")) -> (x*y=w468:dbl[])
        n268 = Array To Cluster(array=w468) -> (cluster=w473:cluster{"[0]":dbl, "[1]":dbl, "[2]":dbl})
        n269 = Array To Cluster(array=w476) -> (cluster=w475:cluster{"[0]":dbl, "[1]":dbl, "[2]":dbl})
        n270 = Array To Cluster(array=w471) -> (cluster=w474:T25)
        n271 = invoke on="Invoke Node" class="SceneGraphDisp (strict)" method="Setup Camera"(reference=w467, "Camera Position"=w473, "Target"=w475, "Up Direction"=w474) -> ()  [unwired: 2 in, 6 out]
      }
      event "Make Awesome Looking": Value Change {
        n272 = event-data() -> ()  [unwired: 1 in, 4 out]
        n273 = control-ref of="Cd Rich Limit"() -> (w490:refnum<vi>)
        n274 = local read "Defect Energy Levels"() -> (w486:cluster{dbl[], dbl[]}[])
        n275 = local read "Cd Rich Limit"() -> (w488:cluster{"appended array":dbl[], dbl[]}[])
        n276 = local read "Te Rich Limit"() -> (w487:cluster{dbl[], dbl[]}[])
        n277 = property on="Defect Energy Levels" class="XYGraph (strict)"() -> ("AnntList"=w485:T26)  [unwired: 2 in, 2 out]
        n278 = Array Size(array=w488) -> (size(s)=w489:i32)
        n279 = for {
          N: w489 -> [_]
          tunnel: w490 -> [w500]
          tunnel: [w498] -> w483 mode=indexing
          tunnel: [w497] -> w484 mode=indexing
          i -> [w499]
          n280 = property on="Property Node" class="XYGraph (strict)"(reference=w500, "Active Plot"=w499) -> ("Plot.Plot Color"=w498:u32, "Plot.Plot Name"=w497:string)  [unwired: 1 in, 2 out]
        }
        n281 = disable-structure shown="Disabled" {
          disable-tunnel: w488 -> [w496 _]
          disable-tunnel: w487 -> [w495 _]
          disable-tunnel: w486 -> [w494 _]
          disable-tunnel: w485 -> [w493 _]
          disable-tunnel: w484 -> [w492 _]
          disable-tunnel: w483 -> [w491 _]
          frame Disabled {
            n282 = call "Awesome Looking Plots for Defect Buddy.vi"("Colors Array"=w491, "Plot Names"=w492, "Annotation List for Charge States"=w493, "Defect Energy Levels"=w494, "Te Rich Limit"=w495, "Cd Rich Limit"=w496) -> ()  [unwired: 6 in]
          }
          frame Enabled {
          }
        }
        n283 = call "Alter Plots for Presentations.vi"("Colors Array"=w483, "Plot Names"=w484, "Annotation List for Charge States"=w485, "Defect Energy Levels"=w486, "Te Rich Limit"=w487, "Cd Rich Limit"=w488) -> ()  [unwired: 6 in]
      }
    }
  }
  n284 = disable-structure shown="Disabled" {
    frame Disabled {
    }
    frame Enabled {
    }
  }
  n285 = disable-structure shown="Disabled" {
    frame Disabled {
      n286 = for {
        N: 9 -> [_]
        i -> [w510]
        n287 = control-ref of="Te Rich Limit"() -> (w504:refnum<vi>)
        n288 = property on="Property Node" class="XYGraph (strict)"(reference=w504, "Active Plot"=w510) -> ("Plot.Point Style"=w509:u8, "Plot.Fill/Pt. Color"=w508:u32, "Plot.Plot Color"=w507:u32, "Plot.Plot Interpolation"=w506:u8, "Plot.Line Width"=w505:u8, "Plot.Line Style"=w502:u8)  [unwired: 1 in, 2 out]
        n289 = control-ref of="Cd Rich Limit"() -> (w503:refnum<vi>)
        n290 = property on="Property Node" class="XYGraph (strict)"(reference=w503, "Active Plot"=w510, "Plot.Point Style"=w509, "Plot.Fill/Pt. Color"=w508, "Plot.Plot Color"=w507, "Plot.Plot Interpolation"=w506, "Plot.Line Width"=w505, "Plot.Line Style"=w502) -> ()  [unwired: 1 in, 2 out]
      }
    }
    frame Enabled {
    }
  }
